vi "MergeMatchPoly.vi"(10 "Poly2D_2":T1, 11 "Poly2D_1":T1) -> (2 "Matched":bool, 3 "Poly2D":T1)   [LabVIEW 2014]
uses:
  TypeDefs/Poly2DwSlope.ctl
  TypeDefs/Point2DwSlope.ctl
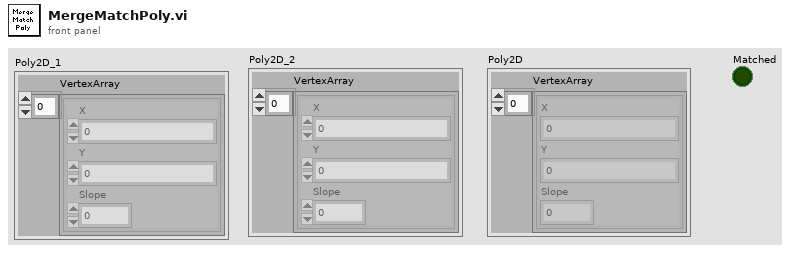
[diagram p1: front panel]
types:
  T1 = typedef "Poly2DwSlope.ctl" = cluster{"VertexArray":T2[]}
  T2 = typedef "Point2DwSlope.ctl" = cluster{"X":sgl, "Y":sgl, "Slope":dbl}
  T3 = enum16{"V1V1", "V1V2", "V2V1", "V2V2", "NoMatch"}
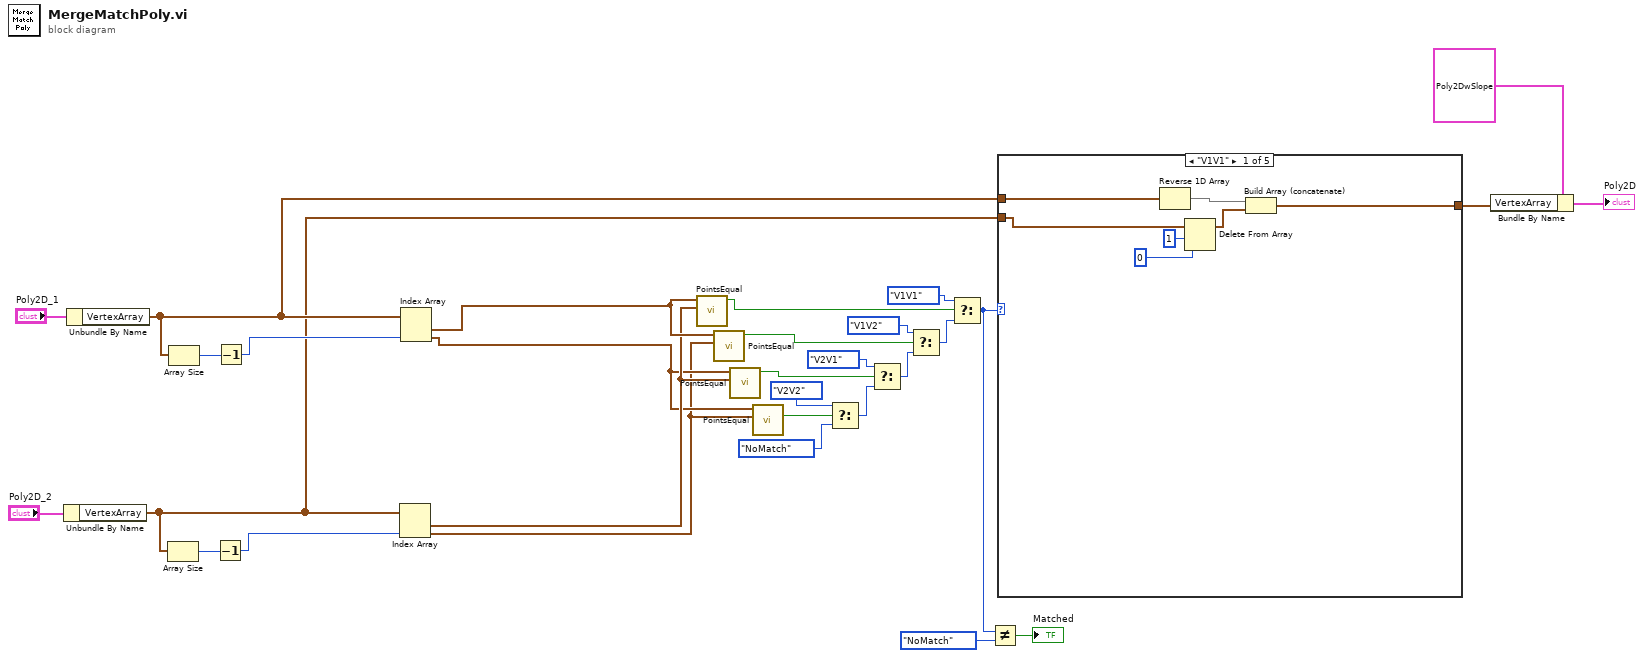
[diagram p0: block diagram]
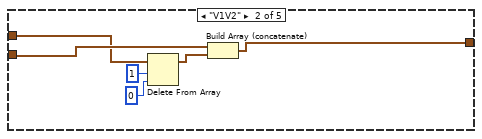
[diagram p2: hidden frame]
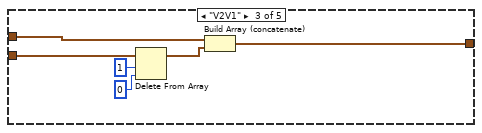
[diagram p3: hidden frame]
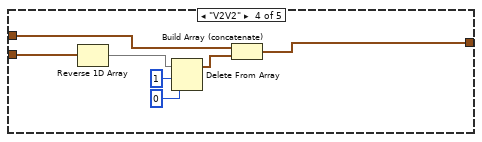
[diagram p4: hidden frame]
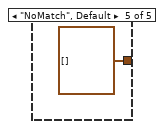
[diagram p5: hidden frame]
diagram:
  n1 = Unbundle By Name("Poly2D_2") -> ("VertexArray"=w12:T2[])
  n2 = Unbundle By Name("Poly2D_1") -> ("VertexArray"=w14:T2[])
  n3 = Array Size(array=w12) -> (size(s)=w27:i32)
  n4 = Array Size(array=w14) -> (size(s)=w30:i32)
  n5 = Decrement(x=w27) -> (x-1=w28:i32)
  n6 = Decrement(x=w30) -> (x-1=w29:i32)
  n7 = Index Array(array=w12, index #2=w28) -> (element #1=w5:T2, element #2=w2:T2)  [unwired: 1 in]
  n8 = Index Array(array=w14, index #2=w29) -> (element #1=w7:T2, element #2=w3:T2)  [unwired: 1 in]
  n9 = call "PointsEqual.vi"("Point2D_2"=w5, "Point2D_1"=w7) -> ("Equal?"=w8:bool)  [unwired: 9 in]
  n10 = call "PointsEqual.vi"("Point2D_2"=w2, "Point2D_1"=w7) -> ("Equal?"=w6:bool)  [unwired: 9 in]
  n11 = call "PointsEqual.vi"("Point2D_2"=w5, "Point2D_1"=w3) -> ("Equal?"=w4:bool)  [unwired: 9 in]
  n12 = call "PointsEqual.vi"("Point2D_2"=w2, "Point2D_1"=w3) -> ("Equal?"=w1:bool)  [unwired: 9 in]
  n13 = Select(t=T3."V2V2" ("f"), s=w1, f=T3."NoMatch") -> (s? t:f=w24:T3)
  n14 = Select(t=T3."V2V1" ("f"), s=w4, f=w24) -> (s? t:f=w25:T3)
  n15 = Select(t=T3."V1V2" ("f"), s=w6, f=w25) -> (s? t:f=w26:T3)
  n16 = Select(t=T3."V1V1" ("f"), s=w8, f=w26) -> (s? t:f=w18:T3)
  n17 = Not Equal?(x=w18, y=T3."NoMatch") -> (x != y?=→"Matched":bool)
  n18 = case shown="\"V1V1\"" w18 {
    tunnel: w14 -> [w37 w41 w49 w55 _]
    tunnel: w12 -> [w33 w42 w47 w56 _]
    tunnel: [w35 w43 w48 w54 T2[] []] -> w10
    frame "V1V1" {
      n19 = Reverse 1D Array(array=w37) -> (reversed array=w36:T2[])
      n20 = Delete From Array(array=w33, length=1, index=0) -> (array with subset deleted=w32:T2[])  [unwired: 1 out]
      n21 = Build Array (concatenate)(w36, w32) -> (w35:T2[])
    }
    frame "V1V2" {
      n22 = Delete From Array(array=w41, length=1, index=0) -> (array with subset deleted=w38:T2[])  [unwired: 1 out]
      n23 = Build Array (concatenate)(w42, w38) -> (w43:T2[])
    }
    frame "V2V1" {
      n24 = Delete From Array(array=w47, length=1, index=0) -> (array with subset deleted=w44:T2[])  [unwired: 1 out]
      n25 = Build Array (concatenate)(w49, w44) -> (w48:T2[])
    }
    frame "V2V2" {
      n26 = Reverse 1D Array(array=w56) -> (reversed array=w53:T2[])
      n27 = Delete From Array(array=w53, length=1, index=0) -> (array with subset deleted=w52:T2[])  [unwired: 1 out]
      n28 = Build Array (concatenate)(w55, w52) -> (w54:T2[])
    }
    frame "NoMatch", Default {
    }
  }
  n29 = Bundle By Name(cluster=T1 {"VertexArray"=[{"X"=8.830601, "Y"=7.172068, "Slope"=0.0}, {"X"=9.048535, "Y"=7.0468507, "Slope"=0.0}, {"X"=7.186762, "Y"=7.89218, "Slope"=0.0}, {"X"=7.186762, "Y"=7.89218, "Slope"=0.0}, {"X"=7.7402935, "Y"=7.713683, "Slope"=0.0}, {"X"=8.830601, "Y"=7.172068, "Slope"=0.0}, {"X"=8.385021, "Y"=7.4258633, "Slope"=0.0}, {"X"=7.7402935, "Y"=7.713683, "Slope"=0.0}, {"X"=9.932331, "Y"=6.418683, "Slope"=0.0}, {"X"=9.839655, "Y"=6.4924364, "Slope"=0.0}, {"X"=9.9016285, "Y"=6.443779, "Slope"=0.0}, {"X"=9.598942, "Y"=6.669884, "Slope"=0.0}, {"X"=9.440515, "Y"=6.776763, "Slope"=0.0}, {"X"=9.048535, "Y"=7.0468507, "Slope"=0.0}, {"X"=8.263897, "Y"=7.4805827, "Slope"=0.0}, {"X"=8.113029, "Y"=7.547746, "Slope"=0.0}, {"X"=8.385021, "Y"=7.4258633, "Slope"=0.0}, {"X"=-0.8597107, "Y"=6.3534126, "Slope"=0.0}, {"X"=-0.7344762, "Y"=6.2797923, "Slope"=0.0}, {"X"=-1.3683765, "Y"=6.656569, "Slope"=0.0}, {"X"=-1.5755129, "Y"=6.777237, "Slope"=0.0}, {"X"=-1.9615697, "Y"=6.9872913, "Slope"=0.0}, {"X"=-0.86309165, "Y"=6.3554897, "Slope"=0.0}, {"X"=0.7361049, "Y"=6.279792, "Slope"=0.0}, {"X"=0.7496544, "Y"=6.2877717, "Slope"=0.0}, {"X"=0.88590366, "Y"=6.367886, "Slope"=0.0}, {"X"=1.1839321, "Y"=6.5489907, "Slope"=0.0}, {"X"=1.7457985, "Y"=6.866745, "Slope"=0.0}, {"X"=1.6707515, "Y"=6.8289485, "Slope"=0.0}, {"X"=1.5142502, "Y"=6.7378664, "Slope"=0.0}, {"X"=1.5142502, "Y"=6.7378664, "Slope"=0.0}, {"X"=1.1839321, "Y"=6.5489907, "Slope"=0.0}, {"X"=0.88590366, "Y"=6.367886, "Slope"=0.0}, {"X"=0.8825039, "Y"=6.3658695, "Slope"=0.0}, {"X"=-9.596155, "Y"=6.670636, "Slope"=0.0}, {"X"=-9.82825, "Y"=6.4999356, "Slope"=0.0}, {"X"=-9.82825, "Y"=6.4999356, "Slope"=0.0}, {"X"=-9.930481, "Y"=6.418602, "Slope"=0.0}, {"X"=-8.38339, "Y"=7.4258623, "Slope"=0.0}, {"X"=-9.046905, "Y"=7.0468526, "Slope"=0.0}, {"X"=-9.439066, "Y"=6.7766366, "Slope"=0.0}, {"X"=-7.7386646, "Y"=7.7136784, "Slope"=0.0}, {"X"=-8.38339, "Y"=7.4258623, "Slope"=0.0}, {"X"=-7.185123, "Y"=7.89218, "Slope"=0.0}, {"X"=-7.439444, "Y"=7.8096337, "Slope"=0.0}, {"X"=-7.2370896, "Y"=7.874528, "Slope"=0.0}, {"X"=-7.113704, "Y"=7.913477, "Slope"=0.0}, {"X"=-7.6962314, "Y"=7.727286, "Slope"=0.0}, {"X"=5.3867097, "Y"=8.087741, "Slope"=0.0}, {"X"=5.732113, "Y"=8.092253, "Slope"=0.0}, {"X"=5.9348326, "Y"=8.090443, "Slope"=0.0}, {"X"=6.061366, "Y"=8.076636, "Slope"=0.0}, {"X"=6.061366, "Y"=8.076636, "Slope"=0.0}, {"X"=2.5593295, "Y"=7.295466, "Slope"=0.0}, {"X"=2.7117634, "Y"=7.365449, "Slope"=0.0}, {"X"=3.1518545, "Y"=7.5595336, "Slope"=0.0}, {"X"=3.387326, "Y"=7.651701, "Slope"=0.0}, {"X"=3.6230888, "Y"=7.737315, "Slope"=0.0}, {"X"=3.6230888, "Y"=7.737315, "Slope"=0.0}, {"X"=4.127137, "Y"=7.8904243, "Slope"=0.0}, {"X"=4.6575503, "Y"=8.007021, "Slope"=0.0}, {"X"=5.21036, "Y"=8.077528, "Slope"=0.0}, {"X"=4.851308, "Y"=8.034141, "Slope"=0.0}, {"X"=3.8247945, "Y"=7.7963767, "Slope"=0.0}, {"X"=4.3288827, "Y"=7.9346447, "Slope"=0.0}, {"X"=6.589266, "Y"=8.020231, "Slope"=0.0}, {"X"=6.589266, "Y"=8.020231, "Slope"=0.0}, {"X"=7.0844173, "Y"=7.9209275, "Slope"=0.0}, {"X"=7.1052027, "Y"=7.9160075, "Slope"=0.0}, {"X"=7.1153355, "Y"=7.9134755, "Slope"=0.0}, {"X"=11.066484, "Y"=5.9259615, "Slope"=0.0}, {"X"=11.296258, "Y"=5.921032, "Slope"=0.0}, {"X"=10.557279, "Y"=6.071126, "Slope"=0.0}, {"X"=10.38447, "Y"=6.147894, "Slope"=0.0}, {"X"=10.217855, "Y"=6.2337523, "Slope"=0.0}, {"X"=10.063343, "Y"=6.3245797, "Slope"=0.0}, {"X"=9.958954, "Y"=6.399936, "Slope"=0.0}, {"X"=11.366602, "Y"=6.3154464, "Slope"=0.0}, {"X"=11.3581505, "Y"=6.325527, "Slope"=0.0}, {"X"=11.381495, "Y"=5.947889, "Slope"=0.0}, {"X"=11.051102, "Y"=5.927362, "Slope"=0.0}, {"X"=11.428065, "Y"=6.2203074, "Slope"=0.0}, {"X"=11.366602, "Y"=6.3154464, "Slope"=0.0}, {"X"=11.4614525, "Y"=6.1327662, "Slope"=0.0}, {"X"=11.428065, "Y"=6.2203074, "Slope"=0.0}, {"X"=11.465086, "Y"=6.056186, "Slope"=0.0}, {"X"=11.4614525, "Y"=6.1327662, "Slope"=0.0}, {"X"=11.438299, "Y"=5.9936595, "Slope"=0.0}, {"X"=11.465086, "Y"=6.056186, "Slope"=0.0}, {"X"=11.438299, "Y"=5.9936595, "Slope"=0.0}, {"X"=11.354124, "Y"=5.938431, "Slope"=0.0}, {"X"=11.296258, "Y"=5.921032, "Slope"=0.0}, {"X"=11.185439, "Y"=5.914531, "Slope"=0.0}, {"X"=11.114248, "Y"=5.9222054, "Slope"=0.0}, {"X"=10.897281, "Y"=5.9582825, "Slope"=0.0}, {"X"=10.843447, "Y"=5.9742303, "Slope"=0.0}, {"X"=10.732583, "Y"=6.0081234, "Slope"=0.0}, {"X"=11.066484, "Y"=5.9259615, "Slope"=0.0}, {"X"=10.732583, "Y"=6.0081234, "Slope"=0.0}, {"X"=10.719951, "Y"=6.0130906, "Slope"=0.0}, {"X"=10.728581, "Y"=6.0096717, "Slope"=0.0}, {"X"=10.450941, "Y"=6.118535, "Slope"=0.0}, {"X"=10.289857, "Y"=6.1987867, "Slope"=0.0}, {"X"=10.174761, "Y"=6.259248, "Slope"=0.0}, {"X"=-0.3831223, "Y"=6.131223, "Slope"=0.0}, {"X"=-0.06600832, "Y"=6.079455, "Slope"=0.0}, {"X"=0.7361049, "Y"=6.279792, "Slope"=0.0}, {"X"=0.49233958, "Y"=6.1676245, "Slope"=0.0}, {"X"=0.41289893, "Y"=6.1388397, "Slope"=0.0}, {"X"=0.34931928, "Y"=6.1239376, "Slope"=0.0}, {"X"=0.06932907, "Y"=6.079732, "Slope"=0.0}, {"X"=0.06932907, "Y"=6.079732, "Slope"=0.0}, {"X"=-0.3457704, "Y"=6.1236205, "Slope"=0.0}, {"X"=-0.7011162, "Y"=6.2621675, "Slope"=0.0}, {"X"=-0.3831223, "Y"=6.131223, "Slope"=0.0}, {"X"=-0.7344762, "Y"=6.2797923, "Slope"=0.0}, {"X"=0.020335363, "Y"=6.074264, "Slope"=0.0}, {"X"=-2.5576975, "Y"=7.295468, "Slope"=0.0}, {"X"=-2.4127276, "Y"=7.2203803, "Slope"=0.0}, {"X"=-2.034087, "Y"=7.027823, "Slope"=0.0}, {"X"=-2.5576975, "Y"=7.295468, "Slope"=0.0}, {"X"=-2.9499915, "Y"=7.4758196, "Slope"=0.0}, {"X"=-2.7095613, "Y"=7.3651953, "Slope"=0.0}, {"X"=-5.784939, "Y"=8.094156, "Slope"=0.0}, {"X"=-5.5782948, "Y"=8.096169, "Slope"=0.0}, {"X"=-5.3852587, "Y"=8.087761, "Slope"=0.0}, {"X"=-5.208071, "Y"=8.077488, "Slope"=0.0}, {"X"=-5.208071, "Y"=8.077488, "Slope"=0.0}, {"X"=-3.3850975, "Y"=7.6514883, "Slope"=0.0}, {"X"=-3.150348, "Y"=7.5595837, "Slope"=0.0}, {"X"=-3.8916922, "Y"=7.821445, "Slope"=0.0}, {"X"=-3.6214588, "Y"=7.73732, "Slope"=0.0}, {"X"=-4.6554594, "Y"=8.006941, "Slope"=0.0}, {"X"=-4.327599, "Y"=7.934705, "Slope"=0.0}, {"X"=-4.1253557, "Y"=7.890371, "Slope"=0.0}, {"X"=-6.50035, "Y"=8.036642, "Slope"=0.0}, {"X"=-6.0605617, "Y"=8.076551, "Slope"=0.0}, {"X"=-5.933233, "Y"=8.090459, "Slope"=0.0}, {"X"=-7.0827866, "Y"=7.9209275, "Slope"=0.0}, {"X"=-6.5884337, "Y"=8.020078, "Slope"=0.0}, {"X"=-7.103572, "Y"=7.916008, "Slope"=0.0}, {"X"=-7.103572, "Y"=7.916008, "Slope"=0.0}, {"X"=1.9629927, "Y"=6.9872847, "Slope"=0.0}, {"X"=2.0286674, "Y"=7.024026, "Slope"=0.0}, {"X"=2.3005672, "Y"=7.166774, "Slope"=0.0}, {"X"=2.4886727, "Y"=7.2611537, "Slope"=0.0}, {"X"=2.5593295, "Y"=7.295466, "Slope"=0.0}, {"X"=2.2341883, "Y"=7.1319356, "Slope"=0.0}, {"X"=-11.046527, "Y"=5.9253874, "Slope"=0.0}, {"X"=-11.183571, "Y"=5.914618, "Slope"=0.0}, {"X"=-11.287836, "Y"=5.9220977, "Slope"=0.0}, {"X"=-10.211346, "Y"=6.231735, "Slope"=0.0}, {"X"=-10.551163, "Y"=6.075544, "Slope"=0.0}, {"X"=-10.033587, "Y"=6.345599, "Slope"=0.0}, {"X"=-10.211346, "Y"=6.231735, "Slope"=0.0}, {"X"=-10.033587, "Y"=6.345599, "Slope"=0.0}, {"X"=-10.060636, "Y"=6.324052, "Slope"=0.0}, {"X"=-11.438604, "Y"=5.9953485, "Slope"=0.0}, {"X"=-11.465441, "Y"=6.0578756, "Slope"=0.0}, {"X"=-11.428589, "Y"=6.222046, "Slope"=0.0}, {"X"=-11.369982, "Y"=6.305766, "Slope"=0.0}, {"X"=-11.363838, "Y"=6.3148956, "Slope"=0.0}, {"X"=-11.336758, "Y"=6.3461637, "Slope"=0.0}, {"X"=-11.306279, "Y"=5.9260035, "Slope"=0.0}, {"X"=-11.38179, "Y"=5.9495883, "Slope"=0.0}, {"X"=-11.417481, "Y"=6.239176, "Slope"=0.0}, {"X"=-11.363838, "Y"=6.3148956, "Slope"=0.0}, {"X"=-11.428589, "Y"=6.222046, "Slope"=0.0}, {"X"=-11.461873, "Y"=6.134476, "Slope"=0.0}, {"X"=-11.46389, "Y"=6.079863, "Slope"=0.0}, {"X"=-11.465441, "Y"=6.0578756, "Slope"=0.0}, {"X"=-11.438604, "Y"=5.9953485, "Slope"=0.0}, {"X"=-11.38179, "Y"=5.9495883, "Slope"=0.0}, {"X"=-11.251305, "Y"=5.9200234, "Slope"=0.0}, {"X"=-11.183571, "Y"=5.914618, "Slope"=0.0}, {"X"=-11.046527, "Y"=5.9253874, "Slope"=0.0}, {"X"=-10.892313, "Y"=5.956102, "Slope"=0.0}, {"X"=-10.892313, "Y"=5.956102, "Slope"=0.0}, {"X"=-10.557951, "Y"=6.072264, "Slope"=0.0}, {"X"=-10.56045, "Y"=6.071302, "Slope"=0.0}, {"X"=-10.727159, "Y"=6.0057144, "Slope"=0.0}, {"X"=-10.379647, "Y"=6.146689, "Slope"=0.0}, {"X"=-10.379647, "Y"=6.146689, "Slope"=0.0}, {"X"=10.444521, "Y"=7.162137, "Slope"=0.0}, {"X"=10.147654, "Y"=7.396959, "Slope"=0.0}, {"X"=11.135348, "Y"=6.5475297, "Slope"=0.0}, {"X"=10.8437395, "Y"=6.8065333, "Slope"=0.0}, {"X"=11.135348, "Y"=6.5475297, "Slope"=0.0}, {"X"=7.7880063, "Y"=8.844079, "Slope"=0.0}, {"X"=9.709546, "Y"=7.7424564, "Slope"=0.0}, {"X"=9.572357, "Y"=7.8359795, "Slope"=0.0}, {"X"=9.48678, "Y"=7.8936634, "Slope"=0.0}, {"X"=9.290509, "Y"=8.026892, "Slope"=0.0}, {"X"=8.41312, "Y"=8.549493, "Slope"=0.0}, {"X"=7.7880063, "Y"=8.844079, "Slope"=0.0}, {"X"=10.147654, "Y"=7.396959, "Slope"=0.0}, {"X"=8.9828415, "Y"=8.233359, "Slope"=0.0}, {"X"=9.290509, "Y"=8.026892, "Slope"=0.0}, {"X"=8.2803135, "Y"=8.623675, "Slope"=0.0}, {"X"=-10.352315, "Y"=7.234274, "Slope"=0.0}, {"X"=-10.44289, "Y"=7.162137, "Slope"=0.0}, {"X"=-9.570726, "Y"=7.8359795, "Slope"=0.0}, {"X"=-9.707915, "Y"=7.7424564, "Slope"=0.0}, {"X"=-10.352315, "Y"=7.234274, "Slope"=0.0}, {"X"=-7.7862473, "Y"=8.8441515, "Slope"=0.0}, {"X"=-8.180492, "Y"=8.666639, "Slope"=0.0}, {"X"=-8.678174, "Y"=8.404416, "Slope"=0.0}, {"X"=-8.24564, "Y"=8.638364, "Slope"=0.0}, {"X"=-8.278681, "Y"=8.623679, "Slope"=0.0}, {"X"=-8.678174, "Y"=8.404416, "Slope"=0.0}, {"X"=-9.570726, "Y"=7.8359795, "Slope"=0.0}, {"X"=-9.404453, "Y"=7.9493356, "Slope"=0.0}, {"X"=-9.108857, "Y"=8.149092, "Slope"=0.0}, {"X"=-9.288878, "Y"=8.026892, "Slope"=0.0}, {"X"=-11.273474, "Y"=6.4113665, "Slope"=0.0}, {"X"=-11.126271, "Y"=6.5544534, "Slope"=0.0}, {"X"=-10.842109, "Y"=6.8065333, "Slope"=0.0}, {"X"=-10.44289, "Y"=7.162137, "Slope"=0.0}, {"X"=-9.838867, "Y"=7.63992, "Slope"=0.0}, {"X"=-9.838867, "Y"=7.63992, "Slope"=0.0}, {"X"=-9.608428, "Y"=7.8105674, "Slope"=0.0}, {"X"=2.3092422, "Y"=9.555755, "Slope"=0.0}, {"X"=6.897631, "Y"=9.15439, "Slope"=0.0}, {"X"=6.9663086, "Y"=9.135237, "Slope"=0.0}, {"X"=6.826199, "Y"=9.173445, "Slope"=0.0}, {"X"=6.826199, "Y"=9.173445, "Slope"=0.0}, {"X"=6.8652363, "Y"=9.162923, "Slope"=0.0}, {"X"=7.4247684, "Y"=8.983244, "Slope"=0.0}, {"X"=7.478522, "Y"=8.961372, "Slope"=0.0}, {"X"=6.9663086, "Y"=9.135237, "Slope"=0.0}, {"X"=7.0981107, "Y"=9.089703, "Slope"=0.0}, {"X"=-7.0928435, "Y"=9.091241, "Slope"=0.0}, {"X"=-7.0928435, "Y"=9.091241, "Slope"=0.0}, {"X"=-7.476928, "Y"=8.961346, "Slope"=0.0}, {"X"=-7.4378753, "Y"=8.977723, "Slope"=0.0}, {"X"=-2.30762, "Y"=9.555743, "Slope"=0.0}, {"X"=-6.9646783, "Y"=9.135236, "Slope"=0.0}, {"X"=-6.8925557, "Y"=9.155159, "Slope"=0.0}, {"X"=6.644459, "Y"=9.217671, "Slope"=0.0}, {"X"=4.169504, "Y"=9.464814, "Slope"=0.0}, {"X"=3.7893963, "Y"=9.464789, "Slope"=0.0}, {"X"=3.404949, "Y"=9.4514675, "Slope"=0.0}, {"X"=5.0040536, "Y"=9.452098, "Slope"=0.0}, {"X"=3.0630891, "Y"=9.468226, "Slope"=0.0}, {"X"=3.0630891, "Y"=9.468226, "Slope"=0.0}, {"X"=2.724652, "Y"=9.495395, "Slope"=0.0}, {"X"=2.8233345, "Y"=9.493452, "Slope"=0.0}, {"X"=5.3548465, "Y"=9.425313, "Slope"=0.0}, {"X"=5.700839, "Y"=9.381838, "Slope"=0.0}, {"X"=6.4296727, "Y"=9.26174, "Slope"=0.0}, {"X"=6.644459, "Y"=9.217671, "Slope"=0.0}, {"X"=6.0274963, "Y"=9.334079, "Slope"=0.0}, {"X"=6.0274963, "Y"=9.334079, "Slope"=0.0}, {"X"=5.7321496, "Y"=9.377271, "Slope"=0.0}, {"X"=5.4556003, "Y"=9.414961, "Slope"=0.0}, {"X"=5.175468, "Y"=9.441919, "Slope"=0.0}, {"X"=4.65047, "Y"=9.461544, "Slope"=0.0}, {"X"=5.0040536, "Y"=9.452098, "Slope"=0.0}, {"X"=4.65047, "Y"=9.461544, "Slope"=0.0}, {"X"=4.607755, "Y"=9.461863, "Slope"=0.0}, {"X"=4.169504, "Y"=9.464814, "Slope"=0.0}, {"X"=3.7893963, "Y"=9.464789, "Slope"=0.0}, {"X"=3.404949, "Y"=9.4514675, "Slope"=0.0}, {"X"=-2.5918474, "Y"=9.499708, "Slope"=0.0}, {"X"=-2.7230513, "Y"=9.495405, "Slope"=0.0}, {"X"=-4.4270477, "Y"=9.454551, "Slope"=0.0}, {"X"=-4.618484, "Y"=9.458359, "Slope"=0.0}, {"X"=-5.072798, "Y"=9.436931, "Slope"=0.0}, {"X"=-6.491574, "Y"=9.240687, "Slope"=0.0}, {"X"=-6.7941, "Y"=9.181162, "Slope"=0.0}, {"X"=-4.618484, "Y"=9.458359, "Slope"=0.0}, {"X"=-3.0264053, "Y"=9.4683485, "Slope"=0.0}, {"X"=-3.0264053, "Y"=9.4683485, "Slope"=0.0}, {"X"=-3.2801545, "Y"=9.449338, "Slope"=0.0}, {"X"=-3.2801545, "Y"=9.449338, "Slope"=0.0}, {"X"=-3.5855074, "Y"=9.461267, "Slope"=0.0}, {"X"=-3.3309553, "Y"=9.444425, "Slope"=0.0}, {"X"=-3.9134116, "Y"=9.468681, "Slope"=0.0}, {"X"=-3.6864495, "Y"=9.468745, "Slope"=0.0}, {"X"=-4.239195, "Y"=9.465216, "Slope"=0.0}, {"X"=-4.1545463, "Y"=9.471141, "Slope"=0.0}, {"X"=-6.2067986, "Y"=9.297449, "Slope"=0.0}, {"X"=-5.920551, "Y"=9.346562, "Slope"=0.0}, {"X"=-5.639876, "Y"=9.383647, "Slope"=0.0}, {"X"=-5.3612723, "Y"=9.4128685, "Slope"=0.0}, {"X"=-5.0972753, "Y"=9.434096, "Slope"=0.0}, {"X"=-4.8120456, "Y"=9.44821, "Slope"=0.0}, {"X"=-6.2067986, "Y"=9.297449, "Slope"=0.0}, {"X"=-5.920551, "Y"=9.346562, "Slope"=0.0}, {"X"=-5.5172114, "Y"=9.401878, "Slope"=0.0}, {"X"=-5.8545833, "Y"=9.354088, "Slope"=0.0}, {"X"=2.2132256, "Y"=9.58271, "Slope"=0.0}, {"X"=1.8189816, "Y"=9.648704, "Slope"=0.0}, {"X"=1.8189816, "Y"=9.648704, "Slope"=0.0}, {"X"=2.2132256, "Y"=9.58271, "Slope"=0.0}, {"X"=-1.6634326, "Y"=9.665585, "Slope"=0.0}, {"X"=-1.8177922, "Y"=9.648689, "Slope"=0.0}, {"X"=-2.2115984, "Y"=9.582698, "Slope"=0.0}, {"X"=-1.9781245, "Y"=9.618462, "Slope"=0.0}, {"X"=0.72814083, "Y"=12.73701, "Slope"=0.0}, {"X"=-0.4196546, "Y"=12.743518, "Slope"=0.0}, {"X"=0.0007652063, "Y"=12.753558, "Slope"=0.0}, {"X"=0.5166687, "Y"=12.742718, "Slope"=0.0}, {"X"=0.4116929, "Y"=12.74487, "Slope"=0.0}, {"X"=1.0176144, "Y"=12.704265, "Slope"=0.0}, {"X"=1.4621797, "Y"=10.655392, "Slope"=0.0}, {"X"=1.5545752, "Y"=9.940707, "Slope"=0.0}, {"X"=1.4498512, "Y"=10.855028, "Slope"=0.0}, {"X"=1.4578543, "Y"=10.732892, "Slope"=0.0}, {"X"=1.5545752, "Y"=9.940707, "Slope"=0.0}, {"X"=1.6384071, "Y"=9.697788, "Slope"=0.0}, {"X"=1.6650634, "Y"=9.665521, "Slope"=0.0}, {"X"=1.5937715, "Y"=9.786305, "Slope"=0.0}, {"X"=1.5833964, "Y"=9.82258, "Slope"=0.0}, {"X"=1.4787083, "Y"=10.454523, "Slope"=0.0}, {"X"=1.4787083, "Y"=10.454523, "Slope"=0.0}, {"X"=1.5225716, "Y"=10.112019, "Slope"=0.0}, {"X"=1.5252, "Y"=10.098917, "Slope"=0.0}, {"X"=1.5426022, "Y"=10.012731, "Slope"=0.0}, {"X"=1.5040516, "Y"=10.237594, "Slope"=0.0}, {"X"=1.4989743, "Y"=10.272214, "Slope"=0.0}, {"X"=-1.6634326, "Y"=9.665585, "Slope"=0.0}, {"X"=-1.6236622, "Y"=9.727999, "Slope"=0.0}, {"X"=-1.5983242, "Y"=9.791381, "Slope"=0.0}, {"X"=-1.552802, "Y"=9.935697, "Slope"=0.0}, {"X"=-1.5983242, "Y"=9.791381, "Slope"=0.0}, {"X"=-1.5869727, "Y"=9.816154, "Slope"=0.0}, {"X"=-1.587823, "Y"=9.813162, "Slope"=0.0}, {"X"=-1.5209501, "Y"=10.100272, "Slope"=0.0}, {"X"=-1.4973384, "Y"=10.267358, "Slope"=0.0}, {"X"=-1.4585742, "Y"=10.705285, "Slope"=0.0}, {"X"=-1.4635025, "Y"=10.629503, "Slope"=0.0}, {"X"=-1.4770607, "Y"=10.45756, "Slope"=0.0}, {"X"=-1.4482204, "Y"=10.855038, "Slope"=0.0}, {"X"=-1.5474311, "Y"=9.963546, "Slope"=0.0}, {"X"=-1.4605238, "Y"=10.667121, "Slope"=0.0}, {"X"=-1.4973384, "Y"=10.267358, "Slope"=0.0}, {"X"=-1.3789781, "Y"=11.701954, "Slope"=0.0}, {"X"=-1.329632, "Y"=12.03006, "Slope"=0.0}, {"X"=-1.4286721, "Y"=11.182402, "Slope"=0.0}, {"X"=-1.0699232, "Y"=12.697788, "Slope"=0.0}, {"X"=-1.0901189, "Y"=12.68052, "Slope"=0.0}, {"X"=-1.1646048, "Y"=12.571568, "Slope"=0.0}, {"X"=-1.2407196, "Y"=12.380032, "Slope"=0.0}, {"X"=-1.2720493, "Y"=12.2814455, "Slope"=0.0}, {"X"=-1.0159835, "Y"=12.704266, "Slope"=0.0}, {"X"=-1.3427985, "Y"=11.95073, "Slope"=0.0}, {"X"=-1.4286721, "Y"=11.182402, "Slope"=0.0}, {"X"=-1.4014932, "Y"=11.485938, "Slope"=0.0}, {"X"=-1.4188328, "Y"=11.319262, "Slope"=0.0}, {"X"=-1.2407196, "Y"=12.380032, "Slope"=0.0}, {"X"=-1.1646048, "Y"=12.571568, "Slope"=0.0}, {"X"=-1.0901189, "Y"=12.68052, "Slope"=0.0}, {"X"=1.1517563, "Y"=12.598272, "Slope"=0.0}, {"X"=1.04348, "Y"=12.704147, "Slope"=0.0}, {"X"=1.0855013, "Y"=12.679428, "Slope"=0.0}, {"X"=1.2149384, "Y"=12.468784, "Slope"=0.0}, {"X"=1.1729327, "Y"=12.554751, "Slope"=0.0}, {"X"=1.1517563, "Y"=12.598272, "Slope"=0.0}, {"X"=1.3806208, "Y"=11.686752, "Slope"=0.0}, {"X"=1.4204677, "Y"=11.315399, "Slope"=0.0}, {"X"=1.4296497, "Y"=11.192336, "Slope"=0.0}, {"X"=1.4498512, "Y"=10.855028, "Slope"=0.0}, {"X"=1.3312752, "Y"=12.016102, "Slope"=0.0}, {"X"=1.3806208, "Y"=11.686752, "Slope"=0.0}, {"X"=1.2736847, "Y"=12.293916, "Slope"=0.0}, {"X"=1.2751907, "Y"=12.2876835, "Slope"=0.0}, {"X"=1.3312752, "Y"=12.016102, "Slope"=0.0}, {"X"=1.2740316, "Y"=12.292477, "Slope"=0.0}, {"X"=1.2736847, "Y"=12.293916, "Slope"=0.0}, {"X"=1.1150376, "Y"=12.643135, "Slope"=0.0}, {"X"=-12.02701, "Y"=-8.883595, "Slope"=0.0}, {"X"=-11.930874, "Y"=-8.755775, "Slope"=0.0}, {"X"=-12.135208, "Y"=-9.147686, "Slope"=0.0}, {"X"=-12.100296, "Y"=-9.031299, "Slope"=0.0}, {"X"=-12.095111, "Y"=-9.902619, "Slope"=0.0}, {"X"=-12.067877, "Y"=-9.970935, "Slope"=0.0}, {"X"=-12.029266, "Y"=-10.067103, "Slope"=0.0}, {"X"=-12.029266, "Y"=-10.067103, "Slope"=0.0}, {"X"=-11.9856825, "Y"=-10.148499, "Slope"=0.0}, {"X"=-12.142309, "Y"=-9.728694, "Slope"=0.0}, {"X"=-12.127801, "Y"=-9.782524, "Slope"=0.0}, {"X"=-12.1486845, "Y"=-9.194613, "Slope"=0.0}, {"X"=-12.170822, "Y"=-9.369725, "Slope"=0.0}, {"X"=-12.1705885, "Y"=-9.389268, "Slope"=0.0}, {"X"=-12.168238, "Y"=-9.549478, "Slope"=0.0}, {"X"=-12.168238, "Y"=-9.549478, "Slope"=0.0}, {"X"=-11.8144655, "Y"=-8.65208, "Slope"=0.0}, {"X"=-11.7577095, "Y"=-8.616993, "Slope"=0.0}, {"X"=-11.8144655, "Y"=-8.65208, "Slope"=0.0}, {"X"=-12.02701, "Y"=-8.883595, "Slope"=0.0}, {"X"=-12.016741, "Y"=-8.869859, "Slope"=0.0}, {"X"=-12.135208, "Y"=-9.147686, "Slope"=0.0}, {"X"=-11.294352, "Y"=-10.777359, "Slope"=0.0}, {"X"=-11.318705, "Y"=-10.768083, "Slope"=0.0}, {"X"=-11.894479, "Y"=-10.297557, "Slope"=0.0}, {"X"=-11.864539, "Y"=-10.3413925, "Slope"=0.0}, {"X"=-11.542754, "Y"=-10.650674, "Slope"=0.0}, {"X"=-11.322815, "Y"=-10.765945, "Slope"=0.0}, {"X"=-11.660817, "Y"=-10.56013, "Slope"=0.0}, {"X"=-11.684228, "Y"=-10.5376215, "Slope"=0.0}, {"X"=-11.768559, "Y"=-10.456095, "Slope"=0.0}, {"X"=-11.768559, "Y"=-10.456095, "Slope"=0.0}, {"X"=-11.318705, "Y"=-10.768083, "Slope"=0.0}, {"X"=-11.864539, "Y"=-10.3413925, "Slope"=0.0}, {"X"=-11.569865, "Y"=-8.037169, "Slope"=0.0}, {"X"=-11.563985, "Y"=-8.070403, "Slope"=0.0}, {"X"=-11.552345, "Y"=-8.164364, "Slope"=0.0}, {"X"=-11.553843, "Y"=-8.257444, "Slope"=0.0}, {"X"=-11.568527, "Y"=-8.345382, "Slope"=0.0}, {"X"=-11.595686, "Y"=-8.425903, "Slope"=0.0}, {"X"=-11.632769, "Y"=-8.4943, "Slope"=0.0}, {"X"=-11.679456, "Y"=-8.552723, "Slope"=0.0}, {"X"=-11.734429, "Y"=-8.599825, "Slope"=0.0}, {"X"=-11.700265, "Y"=-8.574736, "Slope"=0.0}, {"X"=-11.650671, "Y"=-8.521496, "Slope"=0.0}, {"X"=-11.61017, "Y"=-8.45847, "Slope"=0.0}, {"X"=-11.579652, "Y"=-8.387263, "Slope"=0.0}, {"X"=-11.558998, "Y"=-8.305826, "Slope"=0.0}, {"X"=-11.550331, "Y"=-8.218866, "Slope"=0.0}, {"X"=-11.553987, "Y"=-8.128481, "Slope"=0.0}, {"X"=-11.3296585, "Y"=-13.300342, "Slope"=0.0}, {"X"=-11.256834, "Y"=-13.179006, "Slope"=0.0}, {"X"=-11.151226, "Y"=-13.057631, "Slope"=0.0}, {"X"=-11.16577, "Y"=-13.070827, "Slope"=0.0}, {"X"=-11.1825075, "Y"=-13.090706, "Slope"=0.0}, {"X"=-11.051586, "Y"=-12.9728775, "Slope"=0.0}, {"X"=-11.051586, "Y"=-12.9728775, "Slope"=0.0}, {"X"=-10.939525, "Y"=-12.903137, "Slope"=0.0}, {"X"=-10.939525, "Y"=-12.903137, "Slope"=0.0}, {"X"=-10.849801, "Y"=-14.563225, "Slope"=0.0}, {"X"=-11.164953, "Y"=-14.337027, "Slope"=0.0}, {"X"=-11.067114, "Y"=-14.428592, "Slope"=0.0}, {"X"=-11.141206, "Y"=-14.359256, "Slope"=0.0}, {"X"=-11.164953, "Y"=-14.337027, "Slope"=0.0}, {"X"=-10.933373, "Y"=-14.519123, "Slope"=0.0}, {"X"=-10.960547, "Y"=-14.504524, "Slope"=0.0}, {"X"=-11.250185, "Y"=-14.232005, "Slope"=0.0}, {"X"=-11.421939, "Y"=-13.710416, "Slope"=0.0}, {"X"=-11.408769, "Y"=-13.850409, "Slope"=0.0}, {"X"=-11.419471, "Y"=-13.73668, "Slope"=0.0}, {"X"=-11.421939, "Y"=-13.710416, "Slope"=0.0}, {"X"=-11.413157, "Y"=-13.569632, "Slope"=0.0}, {"X"=-11.382209, "Y"=-13.431717, "Slope"=0.0}, {"X"=-11.387743, "Y"=-13.456368, "Slope"=0.0}, {"X"=-11.256834, "Y"=-13.179006, "Slope"=0.0}, {"X"=-11.26992, "Y"=-13.200806, "Slope"=0.0}, {"X"=-11.321019, "Y"=-14.114156, "Slope"=0.0}, {"X"=-11.305685, "Y"=-14.139672, "Slope"=0.0}, {"X"=-11.413157, "Y"=-13.569632, "Slope"=0.0}, {"X"=-11.402093, "Y"=-13.876914, "Slope"=0.0}, {"X"=-11.374592, "Y"=-13.986052, "Slope"=0.0}, {"X"=-11.250185, "Y"=-14.232005, "Slope"=0.0}, {"X"=-11.913404, "Y"=-6.6864777, "Slope"=0.0}, {"X"=-11.797986, "Y"=-7.147725, "Slope"=0.0}, {"X"=-12.13859, "Y"=-5.825948, "Slope"=0.0}, {"X"=-11.913404, "Y"=-6.6864777, "Slope"=0.0}, {"X"=-12.225317, "Y"=-5.519531, "Slope"=0.0}, {"X"=-12.225317, "Y"=-5.519531, "Slope"=0.0}, {"X"=-11.221693, "Y"=-10.810644, "Slope"=0.0}, {"X"=-11.294352, "Y"=-10.777359, "Slope"=0.0}, {"X"=-11.030285, "Y"=-10.970268, "Slope"=0.0}, {"X"=-11.091174, "Y"=-10.905559, "Slope"=0.0}, {"X"=-11.160064, "Y"=-10.849495, "Slope"=0.0}, {"X"=-11.152487, "Y"=-10.854256, "Slope"=0.0}, {"X"=-10.860488, "Y"=-11.333081, "Slope"=0.0}, {"X"=-10.880931, "Y"=-11.255504, "Slope"=0.0}, {"X"=-10.892451, "Y"=-11.2184515, "Slope"=0.0}, {"X"=-10.922376, "Y"=-11.142319, "Slope"=0.0}, {"X"=-10.928037, "Y"=-11.131481, "Slope"=0.0}, {"X"=-10.928037, "Y"=-11.131481, "Slope"=0.0}, {"X"=-10.970161, "Y"=-11.053841, "Slope"=0.0}, {"X"=-11.02817, "Y"=-10.972571, "Slope"=0.0}, {"X"=-10.973595, "Y"=-11.048819, "Slope"=0.0}, {"X"=-11.028286, "Y"=-10.97244, "Slope"=0.0}, {"X"=-11.087512, "Y"=-10.908614, "Slope"=0.0}, {"X"=-10.665473, "Y"=-12.46586, "Slope"=0.0}, {"X"=-10.664033, "Y"=-12.508651, "Slope"=0.0}, {"X"=-10.673386, "Y"=-12.582449, "Slope"=0.0}, {"X"=-10.694738, "Y"=-12.653376, "Slope"=0.0}, {"X"=-10.72751, "Y"=-12.7196455, "Slope"=0.0}, {"X"=-10.768068, "Y"=-12.776132, "Slope"=0.0}, {"X"=-10.816997, "Y"=-12.825721, "Slope"=0.0}, {"X"=-10.902442, "Y"=-12.882612, "Slope"=0.0}, {"X"=-10.916191, "Y"=-12.891214, "Slope"=0.0}, {"X"=-10.800756, "Y"=-12.811512, "Slope"=0.0}, {"X"=-10.754254, "Y"=-12.759442, "Slope"=0.0}, {"X"=-10.716546, "Y"=-12.700924, "Slope"=0.0}, {"X"=-10.686941, "Y"=-12.633139, "Slope"=0.0}, {"X"=-10.668956, "Y"=-12.561274, "Slope"=0.0}, {"X"=-10.663047, "Y"=-12.487158, "Slope"=0.0}, {"X"=-10.665473, "Y"=-12.46586, "Slope"=0.0}, {"X"=-10.710455, "Y"=-14.615379, "Slope"=0.0}, {"X"=-10.849801, "Y"=-14.563225, "Slope"=0.0}, {"X"=-10.848216, "Y"=-14.563806, "Slope"=0.0}, {"X"=-10.7669525, "Y"=-14.595915, "Slope"=0.0}, {"X"=-10.30013, "Y"=-14.642541, "Slope"=0.0}, {"X"=-10.446137, "Y"=-14.654243, "Slope"=0.0}, {"X"=-10.446137, "Y"=-14.654243, "Slope"=0.0}, {"X"=-10.563266, "Y"=-14.646091, "Slope"=0.0}, {"X"=-10.469295, "Y"=-14.651767, "Slope"=0.0}, {"X"=-9.648653, "Y"=-14.927292, "Slope"=0.0}, {"X"=-9.645592, "Y"=-14.928906, "Slope"=0.0}, {"X"=-9.606909, "Y"=-14.948134, "Slope"=0.0}, {"X"=-9.606909, "Y"=-14.948134, "Slope"=0.0}, {"X"=-9.846963, "Y"=-14.788051, "Slope"=0.0}, {"X"=-9.851051, "Y"=-14.785206, "Slope"=0.0}, {"X"=-9.854066, "Y"=-14.783052, "Slope"=0.0}, {"X"=-9.772256, "Y"=-14.849932, "Slope"=0.0}, {"X"=-9.772256, "Y"=-14.849932, "Slope"=0.0}, {"X"=-9.739692, "Y"=-14.872915, "Slope"=0.0}, {"X"=-9.722611, "Y"=-14.884181, "Slope"=0.0}, {"X"=-9.722611, "Y"=-14.884181, "Slope"=0.0}, {"X"=-9.686776, "Y"=-14.906165, "Slope"=0.0}, {"X"=-12.650918, "Y"=-3.9329345, "Slope"=0.0}, {"X"=-12.648346, "Y"=-3.8170426, "Slope"=0.0}, {"X"=-12.631214, "Y"=-3.735219, "Slope"=0.0}, {"X"=-12.623239, "Y"=-3.7092106, "Slope"=0.0}, {"X"=-12.623239, "Y"=-3.7092106, "Slope"=0.0}, {"X"=-12.62978, "Y"=-4.049288, "Slope"=0.0}, {"X"=-12.650918, "Y"=-3.9329345, "Slope"=0.0}, {"X"=-12.57752, "Y"=-3.6137216, "Slope"=0.0}, {"X"=-12.57752, "Y"=-3.6137216, "Slope"=0.0}, {"X"=-12.513479, "Y"=-3.534193, "Slope"=0.0}, {"X"=-12.513479, "Y"=-3.534193, "Slope"=0.0}, {"X"=-12.433673, "Y"=-3.4738154, "Slope"=0.0}, {"X"=-12.433673, "Y"=-3.4738154, "Slope"=0.0}, {"X"=-12.357601, "Y"=-3.4377882, "Slope"=0.0}, {"X"=-12.340974, "Y"=-3.43551, "Slope"=0.0}, {"X"=-3.3543682, "Y"=-1.112888, "Slope"=0.0}, {"X"=-3.2291064, "Y"=-0.992266, "Slope"=0.0}, {"X"=-2.9242365, "Y"=-0.58080864, "Slope"=0.0}, {"X"=-3.0170414, "Y"=-0.7281756, "Slope"=0.0}, {"X"=-3.2999249, "Y"=-1.0642368, "Slope"=0.0}, {"X"=-3.4399374, "Y"=-1.1873536, "Slope"=0.0}, {"X"=-3.0855627, "Y"=-0.82208127, "Slope"=0.0}, {"X"=-3.0855627, "Y"=-0.82208127, "Slope"=0.0}, {"X"=-10.675578, "Y"=-12.364202, "Slope"=0.0}, {"X"=-10.771004, "Y"=-11.824437, "Slope"=0.0}, {"X"=-10.784014, "Y"=-11.759393, "Slope"=0.0}, {"X"=-10.784014, "Y"=-11.759393, "Slope"=0.0}, {"X"=-5.6554403, "Y"=5.9907885, "Slope"=0.0}, {"X"=-4.815982, "Y"=7.0489526, "Slope"=0.0}, {"X"=-4.849929, "Y"=6.9179187, "Slope"=0.0}, {"X"=-5.0451655, "Y"=6.464496, "Slope"=0.0}, {"X"=-5.2916584, "Y"=6.1826806, "Slope"=0.0}, {"X"=-5.162795, "Y"=6.294174, "Slope"=0.0}, {"X"=-5.543999, "Y"=6.0281105, "Slope"=0.0}, {"X"=-6.3306594, "Y"=6.0232587, "Slope"=0.0}, {"X"=-6.6277933, "Y"=6.1670747, "Slope"=0.0}, {"X"=-6.934379, "Y"=6.406201, "Slope"=0.0}, {"X"=-6.8160934, "Y"=6.3108954, "Slope"=0.0}, {"X"=-6.4554677, "Y"=6.0813403, "Slope"=0.0}, {"X"=-6.3306594, "Y"=6.0232587, "Slope"=0.0}, {"X"=-6.250035, "Y"=6.003523, "Slope"=0.0}, {"X"=-5.8642983, "Y"=5.95157, "Slope"=0.0}, {"X"=-5.6554403, "Y"=5.9907885, "Slope"=0.0}, {"X"=-5.924631, "Y"=5.951281, "Slope"=0.0}, {"X"=-4.849929, "Y"=6.9179187, "Slope"=0.0}, {"X"=-5.0451655, "Y"=6.464496, "Slope"=0.0}, {"X"=-10.292118, "Y"=-14.642107, "Slope"=0.0}, {"X"=-10.171297, "Y"=-14.638529, "Slope"=0.0}, {"X"=-10.041175, "Y"=-14.666001, "Slope"=0.0}, {"X"=-10.041588, "Y"=-14.665805, "Slope"=0.0}, {"X"=-10.162641, "Y"=-14.639628, "Slope"=0.0}, {"X"=-10.162641, "Y"=-14.639628, "Slope"=0.0}, {"X"=-10.164488, "Y"=-14.639059, "Slope"=0.0}, {"X"=-10.166433, "Y"=-14.638672, "Slope"=0.0}, {"X"=-9.460867, "Y"=-15.017409, "Slope"=0.0}, {"X"=-9.437974, "Y"=-15.031419, "Slope"=0.0}, {"X"=-9.437974, "Y"=-15.031419, "Slope"=0.0}, {"X"=-9.564893, "Y"=-14.966767, "Slope"=0.0}, {"X"=-9.525483, "Y"=-14.983645, "Slope"=0.0}, {"X"=-9.505892, "Y"=-14.993372, "Slope"=0.0}, {"X"=-9.58607, "Y"=-14.956815, "Slope"=0.0}, {"X"=-9.854066, "Y"=-14.783052, "Slope"=0.0}, {"X"=-9.884875, "Y"=-14.755914, "Slope"=0.0}, {"X"=-9.887594, "Y"=-14.7537775, "Slope"=0.0}, {"X"=-9.901564, "Y"=-14.742871, "Slope"=0.0}, {"X"=-9.548078, "Y"=-14.973137, "Slope"=0.0}, {"X"=-3.9709668, "Y"=0.83104026, "Slope"=0.0}, {"X"=-3.793563, "Y"=0.96303296, "Slope"=0.0}, {"X"=-3.6569257, "Y"=1.1055839, "Slope"=0.0}, {"X"=-3.5894172, "Y"=1.7002168, "Slope"=0.0}, {"X"=-6.403721, "Y"=1.1754698, "Slope"=0.0}, {"X"=-6.3508883, "Y"=1.1123196, "Slope"=0.0}, {"X"=-6.3508883, "Y"=1.1123196, "Slope"=0.0}, {"X"=-3.8743422, "Y"=0.89098823, "Slope"=0.0}, {"X"=-3.673383, "Y"=1.0765003, "Slope"=0.0}, {"X"=-4.5997987, "Y"=2.4074922, "Slope"=0.0}, {"X"=-4.870421, "Y"=2.4419749, "Slope"=0.0}, {"X"=-5.4179683, "Y"=2.447132, "Slope"=0.0}, {"X"=-5.843843, "Y"=2.364739, "Slope"=0.0}, {"X"=-6.137103, "Y"=2.2173433, "Slope"=0.0}, {"X"=-4.5921416, "Y"=0.6193031, "Slope"=0.0}, {"X"=-4.246321, "Y"=0.71311134, "Slope"=0.0}, {"X"=-4.470907, "Y"=0.6456365, "Slope"=0.0}, {"X"=-5.0984373, "Y"=0.6077611, "Slope"=0.0}, {"X"=-5.0984373, "Y"=0.6077611, "Slope"=0.0}, {"X"=-4.658153, "Y"=0.60572743, "Slope"=0.0}, {"X"=-5.2277637, "Y"=0.60893834, "Slope"=0.0}, {"X"=-5.792988, "Y"=0.74757576, "Slope"=0.0}, {"X"=-6.1827035, "Y"=0.97466177, "Slope"=0.0}, {"X"=-4.0832763, "Y"=0.7651222, "Slope"=0.0}, {"X"=-3.5581236, "Y"=1.3308722, "Slope"=0.0}, {"X"=-3.5581236, "Y"=1.3308722, "Slope"=0.0}, {"X"=-3.562323, "Y"=1.6246175, "Slope"=0.0}, {"X"=-6.4372854, "Y"=1.2494335, "Slope"=0.0}, {"X"=-6.532556, "Y"=1.6240577, "Slope"=0.0}, {"X"=-6.472267, "Y"=1.8649976, "Slope"=0.0}, {"X"=-6.358427, "Y"=2.0599158, "Slope"=0.0}, {"X"=-3.5492315, "Y"=1.3571573, "Slope"=0.0}, {"X"=-6.535462, "Y"=1.4654024, "Slope"=0.0}, {"X"=-3.5894172, "Y"=1.7002168, "Slope"=0.0}, {"X"=-6.53032, "Y"=1.7503738, "Slope"=0.0}, {"X"=-4.0369825, "Y"=2.1945257, "Slope"=0.0}, {"X"=-4.0369825, "Y"=2.1945257, "Slope"=0.0}, {"X"=-6.137103, "Y"=2.2173433, "Slope"=0.0}, {"X"=-6.3882627, "Y"=2.0303822, "Slope"=0.0}, {"X"=-4.870421, "Y"=2.4419749, "Slope"=0.0}, {"X"=-5.4179683, "Y"=2.447132, "Slope"=0.0}, {"X"=-5.843843, "Y"=2.364739, "Slope"=0.0}, {"X"=-6.7040663, "Y"=7.639021, "Slope"=0.0}, {"X"=-6.676446, "Y"=7.650669, "Slope"=0.0}, {"X"=-4.9156322, "Y"=7.482542, "Slope"=0.0}, {"X"=-4.855164, "Y"=7.3850617, "Slope"=0.0}, {"X"=-4.815982, "Y"=7.0489526, "Slope"=0.0}, {"X"=-4.8155766, "Y"=7.1894574, "Slope"=0.0}, {"X"=-4.8181634, "Y"=7.2813587, "Slope"=0.0}, {"X"=-5.878805, "Y"=7.82959, "Slope"=0.0}, {"X"=-5.5302444, "Y"=7.8090086, "Slope"=0.0}, {"X"=-5.289001, "Y"=7.740003, "Slope"=0.0}, {"X"=-6.215815, "Y"=7.7961473, "Slope"=0.0}, {"X"=-5.11955, "Y"=7.66165, "Slope"=0.0}, {"X"=-5.0015216, "Y"=7.5747905, "Slope"=0.0}, {"X"=-6.215815, "Y"=7.7961473, "Slope"=0.0}, {"X"=-5.878805, "Y"=7.82959, "Slope"=0.0}, {"X"=-5.5302444, "Y"=7.8090086, "Slope"=0.0}, {"X"=-5.289001, "Y"=7.740003, "Slope"=0.0}, {"X"=-5.0015216, "Y"=7.5747905, "Slope"=0.0}, {"X"=-4.978973, "Y"=7.5499973, "Slope"=0.0}, {"X"=-5.11955, "Y"=7.66165, "Slope"=0.0}, {"X"=-4.855164, "Y"=7.3850617, "Slope"=0.0}, {"X"=-6.8678813, "Y"=7.52537, "Slope"=0.0}, {"X"=-6.777728, "Y"=7.5995193, "Slope"=0.0}, {"X"=-6.856725, "Y"=7.5351534, "Slope"=0.0}, {"X"=-6.8603616, "Y"=7.531958, "Slope"=0.0}, {"X"=-6.875995, "Y"=7.5181913, "Slope"=0.0}, {"X"=-6.888495, "Y"=7.503174, "Slope"=0.0}, {"X"=-6.888495, "Y"=7.503174, "Slope"=0.0}, {"X"=-6.818737, "Y"=7.5675063, "Slope"=0.0}, {"X"=-6.7040663, "Y"=7.639021, "Slope"=0.0}, {"X"=-6.777728, "Y"=7.5995193, "Slope"=0.0}, {"X"=-6.84122, "Y"=7.5485497, "Slope"=0.0}, {"X"=-6.8429217, "Y"=7.5470734, "Slope"=0.0}, {"X"=-6.8310695, "Y"=7.5571713, "Slope"=0.0}, {"X"=-6.875995, "Y"=7.5181913, "Slope"=0.0}, {"X"=-6.8678813, "Y"=7.52537, "Slope"=0.0}, {"X"=-6.818737, "Y"=7.5675063, "Slope"=0.0}, {"X"=-6.822014, "Y"=7.5647697, "Slope"=0.0}, {"X"=-7.0596285, "Y"=6.551442, "Slope"=0.0}, {"X"=-7.091569, "Y"=7.302365, "Slope"=0.0}, {"X"=-7.0596285, "Y"=6.551442, "Slope"=0.0}, {"X"=-7.1912403, "Y"=6.921647, "Slope"=0.0}, {"X"=-7.155486, "Y"=7.136137, "Slope"=0.0}, {"X"=-7.200834, "Y"=7.019425, "Slope"=0.0}, {"X"=-6.894214, "Y"=7.488816, "Slope"=0.0}, {"X"=-7.065946, "Y"=7.3290687, "Slope"=0.0}, {"X"=-7.086213, "Y"=7.308606, "Slope"=0.0}, {"X"=-7.1912403, "Y"=6.921647, "Slope"=0.0}, {"X"=-10.025236, "Y"=-14.673826, "Slope"=0.0}, {"X"=-9.951885, "Y"=-14.708637, "Slope"=0.0}, {"X"=-9.932256, "Y"=-14.721165, "Slope"=0.0}, {"X"=-9.319345, "Y"=-15.105489, "Slope"=0.0}, {"X"=-8.93562, "Y"=-15.3406515, "Slope"=0.0}, {"X"=-9.265467, "Y"=-15.138879, "Slope"=0.0}, {"X"=-9.319345, "Y"=-15.105489, "Slope"=0.0}, {"X"=-8.488454, "Y"=-15.60559, "Slope"=0.0}, {"X"=-8.50379, "Y"=-15.596214, "Slope"=0.0}, {"X"=-8.0269165, "Y"=-15.876325, "Slope"=0.0}, {"X"=-7.546262, "Y"=-16.157545, "Slope"=0.0}, {"X"=-7.6811376, "Y"=-16.072777, "Slope"=0.0}, {"X"=-8.93562, "Y"=-15.3406515, "Slope"=0.0}, {"X"=-8.50379, "Y"=-15.596214, "Slope"=0.0}, {"X"=-8.488454, "Y"=-15.60559, "Slope"=0.0}, {"X"=-7.546262, "Y"=-16.157545, "Slope"=0.0}, {"X"=-7.4288588, "Y"=-16.223211, "Slope"=0.0}, {"X"=-7.2701726, "Y"=-16.31386, "Slope"=0.0}, {"X"=12.028641, "Y"=-8.883595, "Slope"=0.0}, {"X"=11.803545, "Y"=-8.642787, "Slope"=0.0}, {"X"=11.75934, "Y"=-8.616993, "Slope"=0.0}, {"X"=11.932505, "Y"=-8.755775, "Slope"=0.0}, {"X"=11.945703, "Y"=-8.773437, "Slope"=0.0}, {"X"=12.149438, "Y"=-9.191597, "Slope"=0.0}, {"X"=12.150315, "Y"=-9.194613, "Slope"=0.0}, {"X"=12.172453, "Y"=-9.369725, "Slope"=0.0}, {"X"=12.169868, "Y"=-9.549478, "Slope"=0.0}, {"X"=11.987313, "Y"=-10.148499, "Slope"=0.0}, {"X"=12.096742, "Y"=-9.902619, "Slope"=0.0}, {"X"=12.030897, "Y"=-10.067103, "Slope"=0.0}, {"X"=11.987313, "Y"=-10.148499, "Slope"=0.0}, {"X"=12.14394, "Y"=-9.728694, "Slope"=0.0}, {"X"=11.816096, "Y"=-8.65208, "Slope"=0.0}, {"X"=12.028641, "Y"=-8.883595, "Slope"=0.0}, {"X"=12.101927, "Y"=-9.031299, "Slope"=0.0}, {"X"=12.104113, "Y"=-9.038665, "Slope"=0.0}, {"X"=12.136839, "Y"=-9.147686, "Slope"=0.0}, {"X"=12.150315, "Y"=-9.194613, "Slope"=0.0}, {"X"=12.172453, "Y"=-9.369725, "Slope"=0.0}, {"X"=12.169868, "Y"=-9.549478, "Slope"=0.0}, {"X"=12.14394, "Y"=-9.728694, "Slope"=0.0}, {"X"=12.096742, "Y"=-9.902619, "Slope"=0.0}, {"X"=11.571496, "Y"=-8.037169, "Slope"=0.0}, {"X"=11.555617, "Y"=-8.128481, "Slope"=0.0}, {"X"=11.555617, "Y"=-8.128481, "Slope"=0.0}, {"X"=11.551962, "Y"=-8.218866, "Slope"=0.0}, {"X"=11.560629, "Y"=-8.305826, "Slope"=0.0}, {"X"=11.581283, "Y"=-8.387263, "Slope"=0.0}, {"X"=11.611801, "Y"=-8.45847, "Slope"=0.0}, {"X"=11.652302, "Y"=-8.521496, "Slope"=0.0}, {"X"=11.701896, "Y"=-8.574736, "Slope"=0.0}, {"X"=11.73606, "Y"=-8.599825, "Slope"=0.0}, {"X"=11.553976, "Y"=-8.164364, "Slope"=0.0}, {"X"=11.555473, "Y"=-8.257444, "Slope"=0.0}, {"X"=11.570158, "Y"=-8.345382, "Slope"=0.0}, {"X"=11.597317, "Y"=-8.425903, "Slope"=0.0}, {"X"=11.634399, "Y"=-8.4943, "Slope"=0.0}, {"X"=11.681087, "Y"=-8.552723, "Slope"=0.0}, {"X"=11.38384, "Y"=-13.431717, "Slope"=0.0}, {"X"=11.376223, "Y"=-13.986052, "Slope"=0.0}, {"X"=11.32265, "Y"=-14.114156, "Slope"=0.0}, {"X"=10.962178, "Y"=-14.504524, "Slope"=0.0}, {"X"=11.068745, "Y"=-14.428592, "Slope"=0.0}, {"X"=11.166584, "Y"=-14.337027, "Slope"=0.0}, {"X"=11.142837, "Y"=-14.359256, "Slope"=0.0}, {"X"=10.852696, "Y"=-14.562547, "Slope"=0.0}, {"X"=10.906145, "Y"=-14.535062, "Slope"=0.0}, {"X"=10.917822, "Y"=-12.891214, "Slope"=0.0}, {"X"=10.941155, "Y"=-12.903137, "Slope"=0.0}, {"X"=11.053217, "Y"=-12.9728775, "Slope"=0.0}, {"X"=11.152857, "Y"=-13.057631, "Slope"=0.0}, {"X"=11.241991, "Y"=-13.15944, "Slope"=0.0}, {"X"=11.318304, "Y"=-13.278711, "Slope"=0.0}, {"X"=11.3744755, "Y"=-13.408314, "Slope"=0.0}, {"X"=11.331289, "Y"=-13.300342, "Slope"=0.0}, {"X"=10.960146, "Y"=-12.914559, "Slope"=0.0}, {"X"=11.414788, "Y"=-13.569632, "Slope"=0.0}, {"X"=11.152857, "Y"=-13.057631, "Slope"=0.0}, {"X"=11.241991, "Y"=-13.15944, "Slope"=0.0}, {"X"=11.258465, "Y"=-13.179006, "Slope"=0.0}, {"X"=11.414788, "Y"=-13.569632, "Slope"=0.0}, {"X"=11.42357, "Y"=-13.710416, "Slope"=0.0}, {"X"=11.42357, "Y"=-13.710416, "Slope"=0.0}, {"X"=11.410399, "Y"=-13.850409, "Slope"=0.0}, {"X"=11.410399, "Y"=-13.850409, "Slope"=0.0}, {"X"=11.376223, "Y"=-13.986052, "Slope"=0.0}, {"X"=11.32265, "Y"=-14.114156, "Slope"=0.0}, {"X"=11.251816, "Y"=-14.232005, "Slope"=0.0}, {"X"=11.251816, "Y"=-14.232005, "Slope"=0.0}, {"X"=11.068745, "Y"=-14.428592, "Slope"=0.0}, {"X"=10.962178, "Y"=-14.504524, "Slope"=0.0}, {"X"=12.108151, "Y"=-5.9460087, "Slope"=0.0}, {"X"=11.915035, "Y"=-6.6864777, "Slope"=0.0}, {"X"=12.631411, "Y"=-4.049288, "Slope"=0.0}, {"X"=12.463001, "Y"=-4.6658015, "Slope"=0.0}, {"X"=12.140221, "Y"=-5.825948, "Slope"=0.0}, {"X"=12.201659, "Y"=-5.5894847, "Slope"=0.0}, {"X"=11.571496, "Y"=-8.037169, "Slope"=0.0}, {"X"=11.915035, "Y"=-6.6864777, "Slope"=0.0}, {"X"=10.66729, "Y"=-12.416573, "Slope"=0.0}, {"X"=10.664678, "Y"=-12.487158, "Slope"=0.0}, {"X"=10.664678, "Y"=-12.487158, "Slope"=0.0}, {"X"=10.670587, "Y"=-12.561274, "Slope"=0.0}, {"X"=10.688572, "Y"=-12.633139, "Slope"=0.0}, {"X"=10.718177, "Y"=-12.700924, "Slope"=0.0}, {"X"=10.755885, "Y"=-12.759442, "Slope"=0.0}, {"X"=10.802387, "Y"=-12.811512, "Slope"=0.0}, {"X"=10.85663, "Y"=-12.855927, "Slope"=0.0}, {"X"=10.665664, "Y"=-12.508651, "Slope"=0.0}, {"X"=10.675016, "Y"=-12.582449, "Slope"=0.0}, {"X"=10.696369, "Y"=-12.653376, "Slope"=0.0}, {"X"=10.729141, "Y"=-12.7196455, "Slope"=0.0}, {"X"=10.769699, "Y"=-12.776132, "Slope"=0.0}, {"X"=10.917822, "Y"=-12.891214, "Slope"=0.0}, {"X"=10.85663, "Y"=-12.855927, "Slope"=0.0}, {"X"=9.587701, "Y"=-14.956815, "Slope"=0.0}, {"X"=9.648387, "Y"=-14.928349, "Slope"=0.0}, {"X"=9.685769, "Y"=-14.907634, "Slope"=0.0}, {"X"=9.685769, "Y"=-14.907634, "Slope"=0.0}, {"X"=9.706607, "Y"=-14.895271, "Slope"=0.0}, {"X"=9.706607, "Y"=-14.895271, "Slope"=0.0}, {"X"=9.7413225, "Y"=-14.872915, "Slope"=0.0}, {"X"=9.773887, "Y"=-14.849932, "Slope"=0.0}, {"X"=9.789424, "Y"=-14.838251, "Slope"=0.0}, {"X"=9.789424, "Y"=-14.838251, "Slope"=0.0}, {"X"=9.8475485, "Y"=-14.790401, "Slope"=0.0}, {"X"=9.855697, "Y"=-14.783052, "Slope"=0.0}, {"X"=12.5287, "Y"=-3.5463154, "Slope"=0.0}, {"X"=12.579146, "Y"=-3.6137137, "Slope"=0.0}, {"X"=12.590708, "Y"=-3.6321623, "Slope"=0.0}, {"X"=12.590708, "Y"=-3.6321623, "Slope"=0.0}, {"X"=12.3426285, "Y"=-3.4355154, "Slope"=0.0}, {"X"=12.359256, "Y"=-3.4377937, "Slope"=0.0}, {"X"=12.359256, "Y"=-3.4377937, "Slope"=0.0}, {"X"=12.450331, "Y"=-3.4807534, "Slope"=0.0}, {"X"=12.450331, "Y"=-3.4807534, "Slope"=0.0}, {"X"=12.632841, "Y"=-3.7352073, "Slope"=0.0}, {"X"=12.632841, "Y"=-3.7352073, "Slope"=0.0}, {"X"=12.651887, "Y"=-3.8513145, "Slope"=0.0}, {"X"=12.651887, "Y"=-3.8513145, "Slope"=0.0}, {"X"=12.645298, "Y"=-3.9750311, "Slope"=0.0}, {"X"=12.645298, "Y"=-3.9750311, "Slope"=0.0}, {"X"=3.0186722, "Y"=-0.7281756, "Slope"=0.0}, {"X"=2.9258673, "Y"=-0.58080864, "Slope"=0.0}, {"X"=3.2307372, "Y"=-0.992266, "Slope"=0.0}, {"X"=3.0871935, "Y"=-0.82208127, "Slope"=0.0}, {"X"=3.1662605, "Y"=-0.9221965, "Slope"=0.0}, {"X"=3.4415681, "Y"=-1.1873536, "Slope"=0.0}, {"X"=3.355999, "Y"=-1.112888, "Slope"=0.0}, {"X"=3.2307372, "Y"=-0.992266, "Slope"=0.0}, {"X"=10.293746, "Y"=-14.642103, "Slope"=0.0}, {"X"=10.043219, "Y"=-14.665805, "Slope"=0.0}, {"X"=10.042806, "Y"=-14.666001, "Slope"=0.0}, {"X"=10.026867, "Y"=-14.673826, "Slope"=0.0}, {"X"=10.168064, "Y"=-14.638672, "Slope"=0.0}, {"X"=10.166119, "Y"=-14.639059, "Slope"=0.0}, {"X"=10.170087, "Y"=-14.63848, "Slope"=0.0}, {"X"=10.170087, "Y"=-14.63848, "Slope"=0.0}, {"X"=9.889225, "Y"=-14.7537775, "Slope"=0.0}, {"X"=9.886506, "Y"=-14.755914, "Slope"=0.0}, {"X"=9.861074, "Y"=-14.778302, "Slope"=0.0}, {"X"=9.861074, "Y"=-14.778302, "Slope"=0.0}, {"X"=9.566524, "Y"=-14.966767, "Slope"=0.0}, {"X"=9.549708, "Y"=-14.973137, "Slope"=0.0}, {"X"=9.417389, "Y"=-15.04401, "Slope"=0.0}, {"X"=9.439605, "Y"=-15.031419, "Slope"=0.0}, {"X"=9.494886, "Y"=-15.000398, "Slope"=0.0}, {"X"=9.531347, "Y"=-14.98244, "Slope"=0.0}, {"X"=9.507523, "Y"=-14.993372, "Slope"=0.0}, {"X"=9.462498, "Y"=-15.017409, "Slope"=0.0}, {"X"=4.7655854, "Y"=0.60666454, "Slope"=0.0}, {"X"=4.900757, "Y"=2.44138, "Slope"=0.0}, {"X"=4.445768, "Y"=2.35025, "Slope"=0.0}, {"X"=4.0750275, "Y"=2.213103, "Slope"=0.0}, {"X"=4.084907, "Y"=0.7651222, "Slope"=0.0}, {"X"=5.326706, "Y"=0.63066685, "Slope"=0.0}, {"X"=5.719236, "Y"=0.7264725, "Slope"=0.0}, {"X"=5.5209336, "Y"=2.4304006, "Slope"=0.0}, {"X"=3.8698528, "Y"=2.0458076, "Slope"=0.0}, {"X"=3.6970007, "Y"=1.864326, "Slope"=0.0}, {"X"=3.6070752, "Y"=1.2053412, "Slope"=0.0}, {"X"=3.7241516, "Y"=1.0319262, "Slope"=0.0}, {"X"=3.5714078, "Y"=1.6560217, "Slope"=0.0}, {"X"=3.5652642, "Y"=1.6428374, "Slope"=0.0}, {"X"=3.5714078, "Y"=1.6560217, "Slope"=0.0}, {"X"=3.5508623, "Y"=1.3571573, "Slope"=0.0}, {"X"=3.553045, "Y"=1.3868557, "Slope"=0.0}, {"X"=6.3881073, "Y"=1.1548297, "Slope"=0.0}, {"X"=6.4852514, "Y"=1.3510339, "Slope"=0.0}, {"X"=6.5348525, "Y"=1.5920166, "Slope"=0.0}, {"X"=6.4325643, "Y"=1.9461969, "Slope"=0.0}, {"X"=6.002293, "Y"=0.86890256, "Slope"=0.0}, {"X"=6.2358575, "Y"=1.0170529, "Slope"=0.0}, {"X"=6.320571, "Y"=2.0987613, "Slope"=0.0}, {"X"=5.2293944, "Y"=0.60893834, "Slope"=0.0}, {"X"=4.659784, "Y"=0.60572743, "Slope"=0.0}, {"X"=4.659784, "Y"=0.60572743, "Slope"=0.0}, {"X"=5.7946186, "Y"=0.74757576, "Slope"=0.0}, {"X"=5.5763397, "Y"=0.685647, "Slope"=0.0}, {"X"=4.084907, "Y"=0.7651222, "Slope"=0.0}, {"X"=6.352519, "Y"=1.1123196, "Slope"=0.0}, {"X"=6.1843343, "Y"=0.97466177, "Slope"=0.0}, {"X"=3.7241516, "Y"=1.0319262, "Slope"=0.0}, {"X"=6.4053516, "Y"=1.1754698, "Slope"=0.0}, {"X"=6.5370927, "Y"=1.4654024, "Slope"=0.0}, {"X"=6.531951, "Y"=1.7503738, "Slope"=0.0}, {"X"=3.6970007, "Y"=1.864326, "Slope"=0.0}, {"X"=3.8698528, "Y"=2.0458076, "Slope"=0.0}, {"X"=4.1120195, "Y"=2.2329714, "Slope"=0.0}, {"X"=6.3898935, "Y"=2.0303822, "Slope"=0.0}, {"X"=5.740962, "Y"=2.4042594, "Slope"=0.0}, {"X"=5.1689224, "Y"=2.4760795, "Slope"=0.0}, {"X"=4.445768, "Y"=2.35025, "Slope"=0.0}, {"X"=4.6014295, "Y"=2.4074922, "Slope"=0.0}, {"X"=4.8172107, "Y"=7.1894627, "Slope"=0.0}, {"X"=5.491926, "Y"=7.8015456, "Slope"=0.0}, {"X"=5.7070355, "Y"=7.828284, "Slope"=0.0}, {"X"=5.966891, "Y"=7.8276443, "Slope"=0.0}, {"X"=6.2695904, "Y"=7.7851615, "Slope"=0.0}, {"X"=6.6780767, "Y"=7.650669, "Slope"=0.0}, {"X"=6.705697, "Y"=7.639021, "Slope"=0.0}, {"X"=5.022007, "Y"=7.5899568, "Slope"=0.0}, {"X"=4.9459004, "Y"=7.5142617, "Slope"=0.0}, {"X"=4.884291, "Y"=7.4300137, "Slope"=0.0}, {"X"=4.8388834, "Y"=7.3348093, "Slope"=0.0}, {"X"=4.8172107, "Y"=7.1894627, "Slope"=0.0}, {"X"=5.3497233, "Y"=7.7608624, "Slope"=0.0}, {"X"=5.2258754, "Y"=7.7112513, "Slope"=0.0}, {"X"=5.113709, "Y"=7.657008, "Slope"=0.0}, {"X"=5.7070355, "Y"=7.828284, "Slope"=0.0}, {"X"=5.966891, "Y"=7.8276443, "Slope"=0.0}, {"X"=6.2695904, "Y"=7.7851615, "Slope"=0.0}, {"X"=5.022007, "Y"=7.5899568, "Slope"=0.0}, {"X"=5.121181, "Y"=7.66165, "Slope"=0.0}, {"X"=5.0031524, "Y"=7.5747905, "Slope"=0.0}, {"X"=5.2258754, "Y"=7.7112513, "Slope"=0.0}, {"X"=4.8388834, "Y"=7.3348093, "Slope"=0.0}, {"X"=4.884291, "Y"=7.4300137, "Slope"=0.0}, {"X"=5.491926, "Y"=7.8015456, "Slope"=0.0}, {"X"=5.4493246, "Y"=7.7930207, "Slope"=0.0}, {"X"=6.835574, "Y"=7.554695, "Slope"=0.0}, {"X"=6.8738914, "Y"=7.5214505, "Slope"=0.0}, {"X"=6.824801, "Y"=7.5637803, "Slope"=0.0}, {"X"=6.705697, "Y"=7.639021, "Slope"=0.0}, {"X"=6.710484, "Y"=7.6377482, "Slope"=0.0}, {"X"=6.79099, "Y"=7.591445, "Slope"=0.0}, {"X"=6.779359, "Y"=7.5995193, "Slope"=0.0}, {"X"=6.895845, "Y"=7.488816, "Slope"=0.0}, {"X"=6.8901258, "Y"=7.503174, "Slope"=0.0}, {"X"=6.8738914, "Y"=7.5214505, "Slope"=0.0}, {"X"=6.8476286, "Y"=7.5443726, "Slope"=0.0}, {"X"=6.8445525, "Y"=7.5470734, "Slope"=0.0}, {"X"=6.79099, "Y"=7.591445, "Slope"=0.0}, {"X"=6.824801, "Y"=7.5637803, "Slope"=0.0}, {"X"=6.835574, "Y"=7.554695, "Slope"=0.0}, {"X"=6.871907, "Y"=7.523237, "Slope"=0.0}, {"X"=6.864228, "Y"=7.5299687, "Slope"=0.0}, {"X"=7.067577, "Y"=7.3290687, "Slope"=0.0}, {"X"=7.0931997, "Y"=7.302365, "Slope"=0.0}, {"X"=7.006349, "Y"=6.472289, "Slope"=0.0}, {"X"=7.0611887, "Y"=6.5513105, "Slope"=0.0}, {"X"=7.1854534, "Y"=6.8420715, "Slope"=0.0}, {"X"=7.2024646, "Y"=7.019425, "Slope"=0.0}, {"X"=7.067577, "Y"=7.3290687, "Slope"=0.0}, {"X"=7.0931997, "Y"=7.302365, "Slope"=0.0}, {"X"=7.175538, "Y"=6.74118, "Slope"=0.0}, {"X"=9.953516, "Y"=-14.708637, "Slope"=0.0}, {"X"=10.026867, "Y"=-14.673826, "Slope"=0.0}, {"X"=9.903194, "Y"=-14.742871, "Slope"=0.0}, {"X"=9.417389, "Y"=-15.04401, "Slope"=0.0}, {"X"=9.369135, "Y"=-15.07428, "Slope"=0.0}, {"X"=8.505421, "Y"=-15.596214, "Slope"=0.0}, {"X"=8.491675, "Y"=-15.604596, "Slope"=0.0}, {"X"=9.267097, "Y"=-15.138879, "Slope"=0.0}, {"X"=9.267097, "Y"=-15.138879, "Slope"=0.0}, {"X"=8.937251, "Y"=-15.3406515, "Slope"=0.0}, {"X"=8.282294, "Y"=-15.731429, "Slope"=0.0}, {"X"=8.050529, "Y"=-15.86282, "Slope"=0.0}, {"X"=8.069378, "Y"=-15.8505335, "Slope"=0.0}, {"X"=7.6827683, "Y"=-16.072777, "Slope"=0.0}, {"X"=7.5478926, "Y"=-16.157545, "Slope"=0.0}, {"X"=9.187492, "Y"=-15.184627, "Slope"=0.0}, {"X"=8.862729, "Y"=-15.382493, "Slope"=0.0}, {"X"=8.282294, "Y"=-15.731429, "Slope"=0.0}, {"X"=8.4929, "Y"=-15.603772, "Slope"=0.0}, {"X"=7.430489, "Y"=-16.223211, "Slope"=0.0}, {"X"=7.5478926, "Y"=-16.157545, "Slope"=0.0}, {"X"=7.171605, "Y"=-16.371065, "Slope"=0.0}, {"X"=7.171605, "Y"=-16.371065, "Slope"=0.0}, {"X"=11.320335, "Y"=-10.768083, "Slope"=0.0}, {"X"=11.929371, "Y"=-10.2494545, "Slope"=0.0}, {"X"=11.917312, "Y"=-10.265866, "Slope"=0.0}, {"X"=11.885427, "Y"=-10.314343, "Slope"=0.0}, {"X"=11.885427, "Y"=-10.314343, "Slope"=0.0}, {"X"=11.834314, "Y"=-10.379304, "Slope"=0.0}, {"X"=11.74231, "Y"=-10.482889, "Slope"=0.0}, {"X"=11.640282, "Y"=-10.577035, "Slope"=0.0}, {"X"=11.544385, "Y"=-10.650674, "Slope"=0.0}, {"X"=11.86617, "Y"=-10.3413925, "Slope"=0.0}, {"X"=11.295982, "Y"=-10.777359, "Slope"=0.0}, {"X"=11.312095, "Y"=-10.770921, "Slope"=0.0}, {"X"=11.640282, "Y"=-10.577035, "Slope"=0.0}, {"X"=11.74231, "Y"=-10.482889, "Slope"=0.0}, {"X"=11.282086, "Y"=-10.783227, "Slope"=0.0}, {"X"=11.213371, "Y"=-10.816897, "Slope"=0.0}, {"X"=11.14764, "Y"=-10.85966, "Slope"=0.0}, {"X"=11.086128, "Y"=-10.911853, "Slope"=0.0}, {"X"=11.295982, "Y"=-10.777359, "Slope"=0.0}, {"X"=11.029917, "Y"=-10.97244, "Slope"=0.0}, {"X"=10.975225, "Y"=-11.048819, "Slope"=0.0}, {"X"=10.929667, "Y"=-11.131481, "Slope"=0.0}, {"X"=10.894082, "Y"=-11.2184515, "Slope"=0.0}, {"X"=10.870948, "Y"=-11.297758, "Slope"=0.0}, {"X"=10.887574, "Y"=-11.235525, "Slope"=0.0}, {"X"=11.029917, "Y"=-10.97244, "Slope"=0.0}, {"X"=11.0298, "Y"=-10.972571, "Slope"=0.0}, {"X"=10.971792, "Y"=-11.053841, "Slope"=0.0}, {"X"=10.924006, "Y"=-11.142319, "Slope"=0.0}, {"X"=11.086128, "Y"=-10.911853, "Slope"=0.0}, {"X"=11.14764, "Y"=-10.85966, "Slope"=0.0}, {"X"=11.213371, "Y"=-10.816897, "Slope"=0.0}, {"X"=10.301758, "Y"=-14.642538, "Slope"=0.0}, {"X"=10.293746, "Y"=-14.642103, "Slope"=0.0}, {"X"=10.564897, "Y"=-14.646091, "Slope"=0.0}, {"X"=10.851432, "Y"=-14.563225, "Slope"=0.0}, {"X"=10.747182, "Y"=-14.602583, "Slope"=0.0}, {"X"=10.712086, "Y"=-14.615379, "Slope"=0.0}, {"X"=10.564897, "Y"=-14.646091, "Slope"=0.0}, {"X"=10.862119, "Y"=-11.333081, "Slope"=0.0}, {"X"=10.7726345, "Y"=-11.824437, "Slope"=0.0}, {"X"=10.677209, "Y"=-12.364202, "Slope"=0.0}, {"X"=10.66729, "Y"=-12.416573, "Slope"=0.0}, {"X"=4.963912, "Y"=6.637194, "Slope"=0.0}, {"X"=4.8515596, "Y"=6.9179187, "Slope"=0.0}, {"X"=4.8176155, "Y"=7.048952, "Slope"=0.0}, {"X"=5.0467963, "Y"=6.464496, "Slope"=0.0}, {"X"=5.8659306, "Y"=5.9515653, "Slope"=0.0}, {"X"=5.8659306, "Y"=5.9515653, "Slope"=0.0}, {"X"=5.9262633, "Y"=5.951276, "Slope"=0.0}, {"X"=6.33229, "Y"=6.0232587, "Slope"=0.0}, {"X"=6.33229, "Y"=6.0232587, "Slope"=0.0}, {"X"=6.629424, "Y"=6.1670747, "Slope"=0.0}, {"X"=6.629424, "Y"=6.1670747, "Slope"=0.0}, {"X"=6.817724, "Y"=6.3108954, "Slope"=0.0}, {"X"=7.006349, "Y"=6.472289, "Slope"=0.0}, {"X"=5.0467963, "Y"=6.464496, "Slope"=0.0}, {"X"=5.164426, "Y"=6.294174, "Slope"=0.0}, {"X"=5.293289, "Y"=6.1826806, "Slope"=0.0}, {"X"=5.4052844, "Y"=6.1176023, "Slope"=0.0}, {"X"=5.54563, "Y"=6.0281105, "Slope"=0.0}, {"X"=5.54563, "Y"=6.0281105, "Slope"=0.0}, {"X"=5.5747533, "Y"=6.0193143, "Slope"=0.0}, {"X"=-4.928284, "Y"=-17.347603, "Slope"=0.0}, {"X"=-4.485192, "Y"=-17.473867, "Slope"=0.0}, {"X"=-4.0872045, "Y"=-17.574154, "Slope"=0.0}, {"X"=-6.636535, "Y"=-16.656498, "Slope"=0.0}, {"X"=-6.955111, "Y"=-16.489447, "Slope"=0.0}, {"X"=-7.032068, "Y"=-16.445217, "Slope"=0.0}, {"X"=-6.440816, "Y"=-16.758366, "Slope"=0.0}, {"X"=-6.1145263, "Y"=-16.906958, "Slope"=0.0}, {"X"=-6.048642, "Y"=-16.935936, "Slope"=0.0}, {"X"=-5.657333, "Y"=-17.094572, "Slope"=0.0}, {"X"=-4.8739295, "Y"=-17.364567, "Slope"=0.0}, {"X"=-3.6903965, "Y"=-17.662962, "Slope"=0.0}, {"X"=-3.2915175, "Y"=-17.736147, "Slope"=0.0}, {"X"=-5.265338, "Y"=-17.239439, "Slope"=0.0}, {"X"=-6.636535, "Y"=-16.656498, "Slope"=0.0}, {"X"=-6.1145263, "Y"=-16.906958, "Slope"=0.0}, {"X"=-6.3764787, "Y"=-16.788654, "Slope"=0.0}, {"X"=-5.657333, "Y"=-17.094572, "Slope"=0.0}, {"X"=-5.531905, "Y"=-17.140982, "Slope"=0.0}, {"X"=-5.2347617, "Y"=-17.249676, "Slope"=0.0}, {"X"=-4.8739295, "Y"=-17.364567, "Slope"=0.0}, {"X"=-4.485192, "Y"=-17.473867, "Slope"=0.0}, {"X"=-4.0872045, "Y"=-17.574154, "Slope"=0.0}, {"X"=-3.6903965, "Y"=-17.662962, "Slope"=0.0}, {"X"=3.6075315, "Y"=-17.680258, "Slope"=0.0}, {"X"=6.638166, "Y"=-16.656498, "Slope"=0.0}, {"X"=6.781946, "Y"=-16.580774, "Slope"=0.0}, {"X"=6.956742, "Y"=-16.489447, "Slope"=0.0}, {"X"=6.781946, "Y"=-16.580774, "Slope"=0.0}, {"X"=3.6075315, "Y"=-17.680258, "Slope"=0.0}, {"X"=3.7670631, "Y"=-17.646334, "Slope"=0.0}, {"X"=6.2929645, "Y"=-16.828487, "Slope"=0.0}, {"X"=5.9106174, "Y"=-16.992453, "Slope"=0.0}, {"X"=5.3245015, "Y"=-17.21816, "Slope"=0.0}, {"X"=5.133149, "Y"=-17.284317, "Slope"=0.0}, {"X"=4.7839193, "Y"=-17.390415, "Slope"=0.0}, {"X"=3.6920273, "Y"=-17.662962, "Slope"=0.0}, {"X"=6.2929645, "Y"=-16.828487, "Slope"=0.0}, {"X"=6.050273, "Y"=-16.935936, "Slope"=0.0}, {"X"=5.6589637, "Y"=-17.094572, "Slope"=0.0}, {"X"=5.2669687, "Y"=-17.239439, "Slope"=0.0}, {"X"=4.8755603, "Y"=-17.364567, "Slope"=0.0}, {"X"=4.4868226, "Y"=-17.473867, "Slope"=0.0}, {"X"=4.298019, "Y"=-17.521143, "Slope"=0.0}, {"X"=-10.260574, "Y"=-3.3069108, "Slope"=0.0}, {"X"=-11.283855, "Y"=-3.3711903, "Slope"=0.0}, {"X"=-9.970092, "Y"=-3.2923765, "Slope"=0.0}, {"X"=-3.4399374, "Y"=-1.1873536, "Slope"=0.0}, {"X"=-3.521916, "Y"=-1.2533891, "Slope"=0.0}, {"X"=-3.7573729, "Y"=-1.434901, "Slope"=0.0}, {"X"=-3.7573729, "Y"=-1.434901, "Slope"=0.0}, {"X"=-4.0478854, "Y"=-1.6355752, "Slope"=0.0}, {"X"=-4.3772445, "Y"=-1.8462685, "Slope"=0.0}, {"X"=-5.34146, "Y"=-2.3618393, "Slope"=0.0}, {"X"=-5.662619, "Y"=-2.4989357, "Slope"=0.0}, {"X"=-5.024132, "Y"=-2.209944, "Slope"=0.0}, {"X"=-4.7063894, "Y"=-2.058018, "Slope"=0.0}, {"X"=-4.711721, "Y"=-2.061136, "Slope"=0.0}, {"X"=-6.1184225, "Y"=-2.6457238, "Slope"=0.0}, {"X"=-6.607805, "Y"=-2.8040211, "Slope"=0.0}, {"X"=-12.232183, "Y"=-3.4180868, "Slope"=0.0}, {"X"=-12.128426, "Y"=-3.4163973, "Slope"=0.0}, {"X"=-12.232183, "Y"=-3.4180868, "Slope"=0.0}, {"X"=-8.707709, "Y"=-3.1807067, "Slope"=0.0}, {"X"=-9.8188925, "Y"=-3.2787843, "Slope"=0.0}, {"X"=-9.738416, "Y"=-3.2713087, "Slope"=0.0}, {"X"=-9.06884, "Y"=-3.2148187, "Slope"=0.0}, {"X"=-8.707709, "Y"=-3.1807067, "Slope"=0.0}, {"X"=-7.530573, "Y"=-3.0147233, "Slope"=0.0}, {"X"=-11.738921, "Y"=-3.3929737, "Slope"=0.0}, {"X"=-11.843679, "Y"=-3.4006338, "Slope"=0.0}, {"X"=-11.843679, "Y"=-3.4006338, "Slope"=0.0}, {"X"=-10.702967, "Y"=-3.3331478, "Slope"=0.0}, {"X"=-11.072473, "Y"=-3.354675, "Slope"=0.0}, {"X"=-11.1448, "Y"=-3.3608747, "Slope"=0.0}, {"X"=-10.260574, "Y"=-3.3069108, "Slope"=0.0}, {"X"=-11.283855, "Y"=-3.3711903, "Slope"=0.0}, {"X"=-9.380922, "Y"=-3.240731, "Slope"=0.0}, {"X"=-6.607805, "Y"=-2.8040211, "Slope"=0.0}, {"X"=-8.248184, "Y"=-3.1152034, "Slope"=0.0}, {"X"=-7.7203517, "Y"=-3.047589, "Slope"=0.0}, {"X"=-7.119101, "Y"=-2.9200442, "Slope"=0.0}, {"X"=-5.662619, "Y"=-2.4989357, "Slope"=0.0}, {"X"=-6.1184225, "Y"=-2.6457238, "Slope"=0.0}, {"X"=-5.34146, "Y"=-2.3618393, "Slope"=0.0}, {"X"=-5.221523, "Y"=-2.3109796, "Slope"=0.0}, {"X"=-4.0478854, "Y"=-1.6355752, "Slope"=0.0}, {"X"=-4.3772445, "Y"=-1.8462685, "Slope"=0.0}, {"X"=12.233814, "Y"=-3.4180868, "Slope"=0.0}, {"X"=12.130056, "Y"=-3.4163973, "Slope"=0.0}, {"X"=11.893608, "Y"=-3.404276, "Slope"=0.0}, {"X"=11.84531, "Y"=-3.4006338, "Slope"=0.0}, {"X"=9.479367, "Y"=-3.2494392, "Slope"=0.0}, {"X"=11.740552, "Y"=-3.3929737, "Slope"=0.0}, {"X"=7.7219825, "Y"=-3.047589, "Slope"=0.0}, {"X"=5.7348065, "Y"=-2.5273833, "Slope"=0.0}, {"X"=4.692581, "Y"=-2.0487688, "Slope"=0.0}, {"X"=5.2231536, "Y"=-2.3109796, "Slope"=0.0}, {"X"=4.7049255, "Y"=-2.056361, "Slope"=0.0}, {"X"=4.692581, "Y"=-2.0487688, "Slope"=0.0}, {"X"=3.7590036, "Y"=-1.434901, "Slope"=0.0}, {"X"=3.6075091, "Y"=-1.3226423, "Slope"=0.0}, {"X"=3.6075091, "Y"=-1.3226423, "Slope"=0.0}, {"X"=3.4415681, "Y"=-1.1873536, "Slope"=0.0}, {"X"=5.7348065, "Y"=-2.5273833, "Slope"=0.0}, {"X"=10.849632, "Y"=-3.3406618, "Slope"=0.0}, {"X"=11.84531, "Y"=-3.4006338, "Slope"=0.0}, {"X"=11.285486, "Y"=-3.3711903, "Slope"=0.0}, {"X"=10.407241, "Y"=-3.3139515, "Slope"=0.0}, {"X"=9.7400465, "Y"=-3.2713087, "Slope"=0.0}, {"X"=9.479367, "Y"=-3.2494392, "Slope"=0.0}, {"X"=10.407241, "Y"=-3.3139515, "Slope"=0.0}, {"X"=8.70934, "Y"=-3.1807067, "Slope"=0.0}, {"X"=7.7219825, "Y"=-3.047589, "Slope"=0.0}, {"X"=7.5322037, "Y"=-3.0147233, "Slope"=0.0}, {"X"=6.7377086, "Y"=-2.841617, "Slope"=0.0}, {"X"=5.2231536, "Y"=-2.3109796, "Slope"=0.0}, {"X"=4.173215, "Y"=-1.7233979, "Slope"=0.0}, {"X"=2.092016, "Y"=-17.90657, "Slope"=0.0}, {"X"=0.42150292, "Y"=-18.00863, "Slope"=0.0}, {"X"=0.34319338, "Y"=-18.009645, "Slope"=0.0}, {"X"=1.695347, "Y"=-17.944841, "Slope"=0.0}, {"X"=3.1908336, "Y"=-17.753933, "Slope"=0.0}, {"X"=2.9825726, "Y"=-17.7882, "Slope"=0.0}, {"X"=2.7701542, "Y"=-17.82051, "Slope"=0.0}, {"X"=2.5594132, "Y"=-17.850025, "Slope"=0.0}, {"X"=2.490218, "Y"=-17.859251, "Slope"=0.0}, {"X"=3.2931483, "Y"=-17.736147, "Slope"=0.0}, {"X"=2.0012887, "Y"=-17.915014, "Slope"=0.0}, {"X"=2.0012887, "Y"=-17.915014, "Slope"=0.0}, {"X"=0.84556794, "Y"=-17.997324, "Slope"=0.0}, {"X"=0.44709656, "Y"=-18.008022, "Slope"=0.0}, {"X"=0.42150292, "Y"=-18.00863, "Slope"=0.0}, {"X"=1.3231481, "Y"=-17.972385, "Slope"=0.0}, {"X"=1.2700415, "Y"=-17.976114, "Slope"=0.0}, {"X"=2.690039, "Y"=-17.832129, "Slope"=0.0}, {"X"=2.7701542, "Y"=-17.82051, "Slope"=0.0}, {"X"=3.0914207, "Y"=-17.77078, "Slope"=0.0}, {"X"=0.0008154644, "Y"=-18.009115, "Slope"=0.0}, {"X"=-0.0014298288, "Y"=-18.008503, "Slope"=0.0}, {"X"=0.0037170372, "Y"=-18.006178, "Slope"=0.0}, {"X"=0.0030606594, "Y"=-18.008503, "Slope"=0.0}, {"X"=-2.0903852, "Y"=-17.90657, "Slope"=0.0}, {"X"=-3.2915175, "Y"=-17.736147, "Slope"=0.0}, {"X"=-3.1892028, "Y"=-17.753933, "Slope"=0.0}, {"X"=-2.9965718, "Y"=-17.78538, "Slope"=0.0}, {"X"=-2.8064823, "Y"=-17.814571, "Slope"=0.0}, {"X"=-2.616186, "Y"=-17.841745, "Slope"=0.0}, {"X"=-2.3674042, "Y"=-17.87328, "Slope"=0.0}, {"X"=-2.4885871, "Y"=-17.859251, "Slope"=0.0}, {"X"=-0.0020862846, "Y"=-18.006178, "Slope"=0.0}, {"X"=-0.07978936, "Y"=-18.006723, "Slope"=0.0}, {"X"=-0.34159136, "Y"=-18.009645, "Slope"=0.0}, {"X"=-0.8106943, "Y"=-17.998108, "Slope"=0.0}, {"X"=-1.2199664, "Y"=-17.978369, "Slope"=0.0}, {"X"=-1.6231827, "Y"=-17.949776, "Slope"=0.0}, {"X"=-1.6937162, "Y"=-17.944841, "Slope"=0.0}, {"X"=-1.6231827, "Y"=-17.949776, "Slope"=0.0}, {"X"=-2.616186, "Y"=-17.841745, "Slope"=0.0}, {"X"=-2.8064823, "Y"=-17.814571, "Slope"=0.0}, {"X"=-3.0897899, "Y"=-17.77078, "Slope"=0.0}, {"X"=-1.2199664, "Y"=-17.978369, "Slope"=0.0}, {"X"=-0.8106943, "Y"=-17.998108, "Slope"=0.0}, {"X"=-0.00854867, "Y"=3.7263947, "Slope"=0.0}, {"X"=-0.0066404296, "Y"=3.7263823, "Slope"=0.0}, {"X"=0.008271213, "Y"=3.7263823, "Slope"=0.0}, {"X"=-0.76231277, "Y"=2.8479533, "Slope"=0.0}, {"X"=0.6740086, "Y"=2.847094, "Slope"=0.0}, {"X"=0.6740086, "Y"=2.847094, "Slope"=0.0}, {"X"=0.47253898, "Y"=2.847094, "Slope"=0.0}, {"X"=-0.07608838, "Y"=3.7179072, "Slope"=0.0}, {"X"=-0.4628392, "Y"=3.5587547, "Slope"=0.0}, {"X"=-0.3386752, "Y"=3.6528666, "Slope"=0.0}, {"X"=-0.07608838, "Y"=3.7179072, "Slope"=0.0}, {"X"=0.29774323, "Y"=3.670729, "Slope"=0.0}, {"X"=0.34028584, "Y"=3.6528666, "Slope"=0.0}, {"X"=0.46445665, "Y"=3.5587547, "Slope"=0.0}, {"X"=0.060030755, "Y"=3.720132, "Slope"=0.0}, {"X"=0.0101794535, "Y"=3.7263947, "Slope"=0.0}, {"X"=-0.4628392, "Y"=3.5587547, "Slope"=0.0}, {"X"=-0.49247614, "Y"=3.5338767, "Slope"=0.0}, {"X"=-0.49247614, "Y"=3.5338767, "Slope"=0.0}, {"X"=-0.48612607, "Y"=3.5097697, "Slope"=0.0}, {"X"=-0.45324963, "Y"=3.4870713, "Slope"=0.0}, {"X"=-0.39212748, "Y"=3.466576, "Slope"=0.0}, {"X"=-0.49027306, "Y"=3.5230303, "Slope"=0.0}, {"X"=-0.47441077, "Y"=3.5007813, "Slope"=0.0}, {"X"=-0.4386713, "Y"=3.4815457, "Slope"=0.0}, {"X"=-0.3861084, "Y"=3.465226, "Slope"=0.0}, {"X"=-0.24353056, "Y"=3.4534297, "Slope"=0.0}, {"X"=-0.36558542, "Y"=3.4612727, "Slope"=0.0}, {"X"=0.010381071, "Y"=3.4437823, "Slope"=0.0}, {"X"=-0.008876924, "Y"=3.4437895, "Slope"=0.0}, {"X"=-0.008750289, "Y"=3.4437823, "Slope"=0.0}, {"X"=0.010381071, "Y"=3.4437823, "Slope"=0.0}, {"X"=0.48574132, "Y"=3.544352, "Slope"=0.0}, {"X"=0.46445665, "Y"=3.5587547, "Slope"=0.0}, {"X"=0.4877475, "Y"=3.5097704, "Slope"=0.0}, {"X"=0.49189267, "Y"=3.5230253, "Slope"=0.0}, {"X"=0.49409693, "Y"=3.5338771, "Slope"=0.0}, {"X"=0.45487154, "Y"=3.4870725, "Slope"=0.0}, {"X"=0.4760247, "Y"=3.5007768, "Slope"=0.0}, {"X"=0.39375165, "Y"=3.466578, "Slope"=0.0}, {"X"=0.44027802, "Y"=3.4815414, "Slope"=0.0}, {"X"=0.24528153, "Y"=3.4534278, "Slope"=0.0}, {"X"=0.38770628, "Y"=3.465222, "Slope"=0.0}, {"X"=0.0105077075, "Y"=3.4437895, "Slope"=0.0}, {"X"=1.067618, "Y"=2.7614944, "Slope"=0.0}, {"X"=1.0173168, "Y"=2.8046827, "Slope"=0.0}, {"X"=1.0106434, "Y"=2.8081396, "Slope"=0.0}, {"X"=0.998331, "Y"=2.8126178, "Slope"=0.0}, {"X"=0.96865463, "Y"=2.8240356, "Slope"=0.0}, {"X"=0.96865463, "Y"=2.8240356, "Slope"=0.0}, {"X"=1.0473349, "Y"=2.7850795, "Slope"=0.0}, {"X"=1.0565383, "Y"=2.7741954, "Slope"=0.0}, {"X"=0.92898184, "Y"=2.8333485, "Slope"=0.0}, {"X"=0.92898184, "Y"=2.8333485, "Slope"=0.0}, {"X"=0.8959438, "Y"=2.8382154, "Slope"=0.0}, {"X"=0.8375098, "Y"=2.8446708, "Slope"=0.0}, {"X"=0.88944787, "Y"=2.8387268, "Slope"=0.0}, {"X"=0.7639368, "Y"=2.8479538, "Slope"=0.0}, {"X"=-1.045704, "Y"=2.7850792, "Slope"=0.0}, {"X"=-1.0445257, "Y"=2.7859926, "Slope"=0.0}, {"X"=-1.045704, "Y"=2.7850792, "Slope"=0.0}, {"X"=-1.0090119, "Y"=2.8081396, "Slope"=0.0}, {"X"=-0.9670265, "Y"=2.8240356, "Slope"=0.0}, {"X"=-0.8358763, "Y"=2.8446715, "Slope"=0.0}, {"X"=-0.7951621, "Y"=2.8454816, "Slope"=0.0}, {"X"=-0.7951621, "Y"=2.8454816, "Slope"=0.0}, {"X"=-0.8943183, "Y"=2.8382156, "Slope"=0.0}, {"X"=-0.8982203, "Y"=2.8373964, "Slope"=0.0}, {"X"=-0.8982203, "Y"=2.8373964, "Slope"=0.0}, {"X"=-0.9967021, "Y"=2.812618, "Slope"=0.0}, {"X"=-1.0090119, "Y"=2.8081396, "Slope"=0.0}, {"X"=-1.0659869, "Y"=2.7614949, "Slope"=0.0}, {"X"=-1.0549076, "Y"=2.7741952, "Slope"=0.0}, {"X"=-0.48852873, "Y"=2.3884056, "Slope"=0.0}, {"X"=-0.07730713, "Y"=2.3884056, "Slope"=0.0}, {"X"=0.7514543, "Y"=2.386611, "Slope"=0.0}, {"X"=-0.07730713, "Y"=2.3884056, "Slope"=0.0}, {"X"=-1.14167, "Y"=2.3826506, "Slope"=0.0}, {"X"=1.1432979, "Y"=2.3826497, "Slope"=0.0}, {"X"=-0.41324222, "Y"=2.0111115, "Slope"=0.0}, {"X"=-0.70813435, "Y"=2.0103872, "Slope"=0.0}, {"X"=-0.49057758, "Y"=2.0111115, "Slope"=0.0}, {"X"=0.70983547, "Y"=2.0103867, "Slope"=0.0}, {"X"=0.70983547, "Y"=2.0103867, "Slope"=0.0}, {"X"=-0.41324222, "Y"=2.0111115, "Slope"=0.0}, {"X"=1.2337487, "Y"=2.4588747, "Slope"=0.0}, {"X"=1.2165025, "Y"=2.404758, "Slope"=0.0}, {"X"=1.1983142, "Y"=2.397272, "Slope"=0.0}, {"X"=1.1722122, "Y"=2.3927495, "Slope"=0.0}, {"X"=1.1916199, "Y"=2.3954153, "Slope"=0.0}, {"X"=1.1432979, "Y"=2.3826497, "Slope"=0.0}, {"X"=1.2353605, "Y"=2.4271605, "Slope"=0.0}, {"X"=1.228462, "Y"=2.4146354, "Slope"=0.0}, {"X"=1.222558, "Y"=2.4088516, "Slope"=0.0}, {"X"=1.2165025, "Y"=2.404758, "Slope"=0.0}, {"X"=1.226176, "Y"=2.4763017, "Slope"=0.0}, {"X"=1.2289872, "Y"=2.4697802, "Slope"=0.0}, {"X"=1.2092305, "Y"=2.4009252, "Slope"=0.0}, {"X"=1.2353605, "Y"=2.4271605, "Slope"=0.0}, {"X"=1.2364476, "Y"=2.433267, "Slope"=0.0}, {"X"=1.2370933, "Y"=2.441883, "Slope"=0.0}, {"X"=1.4738536, "Y"=2.006581, "Slope"=0.0}, {"X"=1.4669265, "Y"=2.0087044, "Slope"=0.0}, {"X"=1.4593807, "Y"=2.009836, "Slope"=0.0}, {"X"=1.4574188, "Y"=2.009671, "Slope"=0.0}, {"X"=1.5014237, "Y"=1.9812346, "Slope"=0.0}, {"X"=1.4986236, "Y"=1.9855362, "Slope"=0.0}, {"X"=1.4926502, "Y"=1.9933399, "Slope"=0.0}, {"X"=1.4872434, "Y"=1.9984872, "Slope"=0.0}, {"X"=1.4812546, "Y"=2.0027587, "Slope"=0.0}, {"X"=1.4748765, "Y"=2.0060189, "Slope"=0.0}, {"X"=1.4802402, "Y"=2.0035176, "Slope"=0.0}, {"X"=1.4971714, "Y"=1.9878777, "Slope"=0.0}, {"X"=1.4920352, "Y"=1.9941158, "Slope"=0.0}, {"X"=1.4863943, "Y"=1.9993223, "Slope"=0.0}, {"X"=1.4593807, "Y"=2.009836, "Slope"=0.0}, {"X"=1.459968, "Y"=2.0097, "Slope"=0.0}, {"X"=-1.4576082, "Y"=2.009493, "Slope"=0.0}, {"X"=-1.457856, "Y"=2.0095024, "Slope"=0.0}, {"X"=-1.457856, "Y"=2.0095024, "Slope"=0.0}, {"X"=-1.4649794, "Y"=2.008526, "Slope"=0.0}, {"X"=-1.4716955, "Y"=2.0065548, "Slope"=0.0}, {"X"=-1.4780617, "Y"=2.0036175, "Slope"=0.0}, {"X"=-1.4843178, "Y"=1.9994733, "Slope"=0.0}, {"X"=-1.4902166, "Y"=1.9941378, "Slope"=0.0}, {"X"=-1.4956957, "Y"=1.9875569, "Slope"=0.0}, {"X"=-1.4960741, "Y"=1.986977, "Slope"=0.0}, {"X"=-1.4960741, "Y"=1.986977, "Slope"=0.0}, {"X"=-1.4579788, "Y"=2.009514, "Slope"=0.0}, {"X"=-1.4956957, "Y"=1.9875569, "Slope"=0.0}, {"X"=-1.4902166, "Y"=1.9941378, "Slope"=0.0}, {"X"=-1.4843178, "Y"=1.9994733, "Slope"=0.0}, {"X"=-1.4780617, "Y"=2.0036175, "Slope"=0.0}, {"X"=-1.4716955, "Y"=2.0065548, "Slope"=0.0}, {"X"=-1.2316467, "Y"=2.459709, "Slope"=0.0}, {"X"=-1.1959518, "Y"=2.398109, "Slope"=0.0}, {"X"=-1.1960353, "Y"=2.3981266, "Slope"=0.0}, {"X"=-1.2158687, "Y"=2.406542, "Slope"=0.0}, {"X"=-1.2276436, "Y"=2.4172268, "Slope"=0.0}, {"X"=-1.2336802, "Y"=2.4300911, "Slope"=0.0}, {"X"=-1.2346641, "Y"=2.4445548, "Slope"=0.0}, {"X"=-1.2352839, "Y"=2.442157, "Slope"=0.0}, {"X"=-1.1959518, "Y"=2.398109, "Slope"=0.0}, {"X"=-1.1648246, "Y"=2.3918023, "Slope"=0.0}, {"X"=-1.1706961, "Y"=2.3924835, "Slope"=0.0}, {"X"=-1.2245513, "Y"=2.476303, "Slope"=0.0}, {"X"=-1.2336527, "Y"=2.4271784, "Slope"=0.0}, {"X"=-1.2276436, "Y"=2.4172268, "Slope"=0.0}, {"X"=-1.1960255, "Y"=2.398121, "Slope"=0.0}, {"X"=-1.2145584, "Y"=2.405078, "Slope"=0.0}, {"X"=1.5076458, "Y"=1.9700412, "Slope"=0.0}, {"X"=1.78655, "Y"=1.4684, "Slope"=0.0}, {"X"=1.78655, "Y"=1.4684, "Slope"=0.0}, {"X"=1.8523945, "Y"=1.34997, "Slope"=0.0}, {"X"=1.8655576, "Y"=1.3262943, "Slope"=0.0}, {"X"=1.8931534, "Y"=1.2766625, "Slope"=0.0}, {"X"=1.8931534, "Y"=1.2766625, "Slope"=0.0}, {"X"=1.9770744, "Y"=1.1257194, "Slope"=0.0}, {"X"=1.9836459, "Y"=1.1138973, "Slope"=0.0}, {"X"=2.2579062, "Y"=0.62060535, "Slope"=0.0}, {"X"=2.3439512, "Y"=0.4658459, "Slope"=0.0}, {"X"=2.4375534, "Y"=0.29749277, "Slope"=0.0}, {"X"=2.4375534, "Y"=0.29749277, "Slope"=0.0}, {"X"=2.5186753, "Y"=0.151581, "Slope"=0.0}, {"X"=2.6968968, "Y"=-0.16897915, "Slope"=0.0}, {"X"=2.8735185, "Y"=-0.4866523, "Slope"=0.0}, {"X"=2.634508, "Y"=-0.056768816, "Slope"=0.0}, {"X"=2.8530045, "Y"=-0.44975382, "Slope"=0.0}, {"X"=1.1919955, "Y"=2.5377808, "Slope"=0.0}, {"X"=1.1919955, "Y"=2.5377808, "Slope"=0.0}, {"X"=1.5014237, "Y"=1.9812346, "Slope"=0.0}, {"X"=-1.4998013, "Y"=1.9812322, "Slope"=0.0}, {"X"=-1.5060034, "Y"=1.970079, "Slope"=0.0}, {"X"=-1.784904, "Y"=1.4684283, "Slope"=0.0}, {"X"=-1.857495, "Y"=1.3378601, "Slope"=0.0}, {"X"=-1.8507538, "Y"=1.3499885, "Slope"=0.0}, {"X"=-1.2245513, "Y"=2.476303, "Slope"=0.0}, {"X"=-1.0659869, "Y"=2.7614949, "Slope"=0.0}, {"X"=-1.7710594, "Y"=1.4933293, "Slope"=0.0}, {"X"=-1.8639268, "Y"=1.3262943, "Slope"=0.0}, {"X"=-1.8915226, "Y"=1.2766625, "Slope"=0.0}, {"X"=-1.9820136, "Y"=1.113902, "Slope"=0.0}, {"X"=-2.1730704, "Y"=0.7702549, "Slope"=0.0}, {"X"=-2.2562754, "Y"=0.62060535, "Slope"=0.0}, {"X"=-2.4359226, "Y"=0.29749277, "Slope"=0.0}, {"X"=-2.632877, "Y"=-0.056768816, "Slope"=0.0}, {"X"=-2.8513737, "Y"=-0.44975382, "Slope"=0.0}, {"X"=-2.3423204, "Y"=0.4658459, "Slope"=0.0}, {"X"=-2.5170445, "Y"=0.151581, "Slope"=0.0}, {"X"=-2.695266, "Y"=-0.16897915, "Slope"=0.0}, {"X"=-2.8718877, "Y"=-0.4866523, "Slope"=0.0}, {"X"=-1.9754436, "Y"=1.1257194, "Slope"=0.0}, {"X"=-6.1731024, "Y"=0.80225223, "Slope"=0.0}, {"X"=-6.4152503, "Y"=1.0218331, "Slope"=0.0}, {"X"=-6.608058, "Y"=1.2818588, "Slope"=0.0}, {"X"=-6.6882205, "Y"=1.5042956, "Slope"=0.0}, {"X"=-6.6324167, "Y"=1.8278004, "Slope"=0.0}, {"X"=-6.4458513, "Y"=2.1040184, "Slope"=0.0}, {"X"=-6.1973596, "Y"=2.3407633, "Slope"=0.0}, {"X"=-5.523589, "Y"=0.5446353, "Slope"=0.0}, {"X"=-5.79826, "Y"=2.4814765, "Slope"=0.0}, {"X"=-4.867923, "Y"=0.47854578, "Slope"=0.0}, {"X"=-5.3243194, "Y"=2.5744805, "Slope"=0.0}, {"X"=-3.50968, "Y"=1.0301466, "Slope"=0.0}, {"X"=-3.4327807, "Y"=1.2001191, "Slope"=0.0}, {"X"=-3.3941116, "Y"=1.382841, "Slope"=0.0}, {"X"=-3.4603047, "Y"=1.7814922, "Slope"=0.0}, {"X"=-4.809182, "Y"=0.48575115, "Slope"=0.0}, {"X"=-4.405914, "Y"=0.54676175, "Slope"=0.0}, {"X"=-4.595913, "Y"=2.5052567, "Slope"=0.0}, {"X"=-4.0831995, "Y"=0.6346704, "Slope"=0.0}, {"X"=-4.1484256, "Y"=2.3729658, "Slope"=0.0}, {"X"=-3.6613507, "Y"=0.885137, "Slope"=0.0}, {"X"=-3.85941, "Y"=0.7556109, "Slope"=0.0}, {"X"=-4.011697, "Y"=0.66795987, "Slope"=0.0}, {"X"=-6.1973596, "Y"=2.3407633, "Slope"=0.0}, {"X"=-5.79826, "Y"=2.4814765, "Slope"=0.0}, {"X"=-5.3243194, "Y"=2.5744805, "Slope"=0.0}, {"X"=-4.595913, "Y"=2.5052567, "Slope"=0.0}, {"X"=-6.4458513, "Y"=2.1040184, "Slope"=0.0}, {"X"=-3.5067923, "Y"=1.8703905, "Slope"=0.0}, {"X"=-3.5067923, "Y"=1.8703905, "Slope"=0.0}, {"X"=-6.6324167, "Y"=1.8278004, "Slope"=0.0}, {"X"=-3.4603047, "Y"=1.7814922, "Slope"=0.0}, {"X"=-6.6882205, "Y"=1.5042956, "Slope"=0.0}, {"X"=-3.3941116, "Y"=1.382841, "Slope"=0.0}, {"X"=-6.608058, "Y"=1.2818588, "Slope"=0.0}, {"X"=-3.4327807, "Y"=1.2001191, "Slope"=0.0}, {"X"=-6.4152503, "Y"=1.0218331, "Slope"=0.0}, {"X"=-3.50968, "Y"=1.0301466, "Slope"=0.0}, {"X"=-3.5353258, "Y"=0.9944994, "Slope"=0.0}, {"X"=-6.1731024, "Y"=0.80225223, "Slope"=0.0}, {"X"=-3.7040718, "Y"=0.85061496, "Slope"=0.0}, {"X"=-5.523589, "Y"=0.5446353, "Slope"=0.0}, {"X"=-4.405914, "Y"=0.54676175, "Slope"=0.0}, {"X"=-4.809182, "Y"=0.48575115, "Slope"=0.0}, {"X"=-4.1103888, "Y"=2.2329714, "Slope"=0.0}, {"X"=-4.869828, "Y"=2.4418511, "Slope"=0.0}, {"X"=-5.417605, "Y"=2.4471264, "Slope"=0.0}, {"X"=-5.843739, "Y"=2.3647609, "Slope"=0.0}, {"X"=-3.5717738, "Y"=1.6587385, "Slope"=0.0}, {"X"=-5.717605, "Y"=0.7264725, "Slope"=0.0}, {"X"=-6.403721, "Y"=1.1754698, "Slope"=0.0}, {"X"=-4.0733967, "Y"=2.213103, "Slope"=0.0}, {"X"=-4.0369825, "Y"=2.1945257, "Slope"=0.0}, {"X"=-3.8689134, "Y"=2.0467944, "Slope"=0.0}, {"X"=-3.8689134, "Y"=2.0467944, "Slope"=0.0}, {"X"=-3.695971, "Y"=1.8667909, "Slope"=0.0}, {"X"=-3.7373013, "Y"=1.9342899, "Slope"=0.0}, {"X"=-3.5643377, "Y"=1.6428626, "Slope"=0.0}, {"X"=-5.574709, "Y"=0.685647, "Slope"=0.0}, {"X"=-3.5498102, "Y"=1.3571969, "Slope"=0.0}, {"X"=-3.6723025, "Y"=1.0764607, "Slope"=0.0}, {"X"=-4.7639546, "Y"=0.60666454, "Slope"=0.0}, {"X"=-3.873783, "Y"=0.89096785, "Slope"=0.0}, {"X"=-4.470907, "Y"=0.6456365, "Slope"=0.0}, {"X"=-5.7393327, "Y"=2.4042227, "Slope"=0.0}, {"X"=-4.869828, "Y"=2.4418511, "Slope"=0.0}, {"X"=-5.417605, "Y"=2.4471264, "Slope"=0.0}, {"X"=-6.31894, "Y"=2.0987613, "Slope"=0.0}, {"X"=-6.31894, "Y"=2.0987613, "Slope"=0.0}, {"X"=-3.5643377, "Y"=1.6428626, "Slope"=0.0}, {"X"=-6.1827035, "Y"=0.97466177, "Slope"=0.0}, {"X"=-6.53032, "Y"=1.7503738, "Slope"=0.0}, {"X"=-6.3882627, "Y"=2.0303822, "Slope"=0.0}, {"X"=-3.5498102, "Y"=1.3571969, "Slope"=0.0}, {"X"=-6.5354886, "Y"=1.4654716, "Slope"=0.0}, {"X"=-6.53032, "Y"=1.7503738, "Slope"=0.0}, {"X"=-3.6723025, "Y"=1.0764607, "Slope"=0.0}, {"X"=-6.2342267, "Y"=1.0170529, "Slope"=0.0}, {"X"=-6.1827035, "Y"=0.97466177, "Slope"=0.0}, {"X"=-6.483632, "Y"=1.3510634, "Slope"=0.0}, {"X"=-3.717171, "Y"=1.0358701, "Slope"=0.0}, {"X"=-6.403721, "Y"=1.1754698, "Slope"=0.0}, {"X"=-6.3864765, "Y"=1.1548297, "Slope"=0.0}, {"X"=-6.0006623, "Y"=0.86890256, "Slope"=0.0}, {"X"=-5.574709, "Y"=0.685647, "Slope"=0.0}, {"X"=-4.470907, "Y"=0.6456365, "Slope"=0.0}, {"X"=-4.7639546, "Y"=0.60666454, "Slope"=0.0}, {"X"=-5.325075, "Y"=0.63066685, "Slope"=0.0}, {"X"=5.768352, "Y"=2.4869251, "Slope"=0.0}, {"X"=6.256812, "Y"=2.3057399, "Slope"=0.0}, {"X"=3.3904872, "Y"=1.4368991, "Slope"=0.0}, {"X"=6.115471, "Y"=0.7700497, "Slope"=0.0}, {"X"=4.9278536, "Y"=2.5646243, "Slope"=0.0}, {"X"=6.607655, "Y"=1.9358124, "Slope"=0.0}, {"X"=4.4356084, "Y"=2.454596, "Slope"=0.0}, {"X"=6.7040563, "Y"=1.5566156, "Slope"=0.0}, {"X"=4.024505, "Y"=2.3008115, "Slope"=0.0}, {"X"=6.6571274, "Y"=1.3635727, "Slope"=0.0}, {"X"=3.8814108, "Y"=2.2197797, "Slope"=0.0}, {"X"=6.5468025, "Y"=1.168247, "Slope"=0.0}, {"X"=3.4867268, "Y"=1.8398644, "Slope"=0.0}, {"X"=6.373358, "Y"=0.9706594, "Slope"=0.0}, {"X"=3.418811, "Y"=1.2466412, "Slope"=0.0}, {"X"=5.567228, "Y"=0.5589959, "Slope"=0.0}, {"X"=3.4960277, "Y"=1.0581442, "Slope"=0.0}, {"X"=3.6728444, "Y"=0.8732367, "Slope"=0.0}, {"X"=5.017665, "Y"=0.49480686, "Slope"=0.0}, {"X"=3.9657695, "Y"=0.6925165, "Slope"=0.0}, {"X"=4.5461817, "Y"=0.5221703, "Slope"=0.0}, {"X"=6.3164315, "Y"=0.9224521, "Slope"=0.0}, {"X"=3.474629, "Y"=1.8224995, "Slope"=0.0}, {"X"=3.4075844, "Y"=1.5070968, "Slope"=0.0}, {"X"=3.3904872, "Y"=1.4368991, "Slope"=0.0}, {"X"=5.517816, "Y"=0.5428311, "Slope"=0.0}, {"X"=4.866611, "Y"=0.4799412, "Slope"=0.0}, {"X"=5.567228, "Y"=0.5589959, "Slope"=0.0}, {"X"=4.210116, "Y"=0.57917607, "Slope"=0.0}, {"X"=6.115471, "Y"=0.7700497, "Slope"=0.0}, {"X"=6.1346426, "Y"=0.7791764, "Slope"=0.0}, {"X"=3.9657695, "Y"=0.6925165, "Slope"=0.0}, {"X"=6.373358, "Y"=0.9706594, "Slope"=0.0}, {"X"=3.543388, "Y"=0.9885701, "Slope"=0.0}, {"X"=6.5468025, "Y"=1.168247, "Slope"=0.0}, {"X"=3.4960277, "Y"=1.0581442, "Slope"=0.0}, {"X"=6.6571274, "Y"=1.3635727, "Slope"=0.0}, {"X"=3.418811, "Y"=1.2466412, "Slope"=0.0}, {"X"=6.7040563, "Y"=1.5566156, "Slope"=0.0}, {"X"=6.607655, "Y"=1.9358124, "Slope"=0.0}, {"X"=3.514335, "Y"=1.8804414, "Slope"=0.0}, {"X"=6.111094, "Y"=2.3925397, "Slope"=0.0}, {"X"=5.4517217, "Y"=2.575982, "Slope"=0.0}, {"X"=4.7988167, "Y"=2.5636787, "Slope"=0.0}, {"X"=4.1516795, "Y"=2.3743773, "Slope"=0.0}, {"X"=3.8814108, "Y"=2.2197797, "Slope"=0.0}, {"X"=3.9731412, "Y"=0.83052903, "Slope"=0.0}, {"X"=3.795828, "Y"=0.9617485, "Slope"=0.0}, {"X"=3.6591375, "Y"=1.1025287, "Slope"=0.0}, {"X"=3.5967474, "Y"=1.7109286, "Slope"=0.0}, {"X"=4.601434, "Y"=2.407352, "Slope"=0.0}, {"X"=4.247952, "Y"=0.71311134, "Slope"=0.0}, {"X"=4.5937724, "Y"=0.6193031, "Slope"=0.0}, {"X"=6.360058, "Y"=2.0599158, "Slope"=0.0}, {"X"=6.473898, "Y"=1.8649976, "Slope"=0.0}, {"X"=6.534187, "Y"=1.6240577, "Slope"=0.0}, {"X"=6.438916, "Y"=1.2494335, "Slope"=0.0}, {"X"=6.352519, "Y"=1.1123196, "Slope"=0.0}, {"X"=6.1843343, "Y"=0.97466177, "Slope"=0.0}, {"X"=5.7946186, "Y"=0.74757576, "Slope"=0.0}, {"X"=5.7946186, "Y"=0.74757576, "Slope"=0.0}, {"X"=6.473898, "Y"=1.8649976, "Slope"=0.0}, {"X"=4.8706145, "Y"=2.4416611, "Slope"=0.0}, {"X"=5.4187417, "Y"=2.447126, "Slope"=0.0}, {"X"=5.100068, "Y"=0.6077611, "Slope"=0.0}, {"X"=5.2293944, "Y"=0.60893834, "Slope"=0.0}, {"X"=5.5763397, "Y"=0.685647, "Slope"=0.0}, {"X"=4.5937724, "Y"=0.6193031, "Slope"=0.0}, {"X"=4.247952, "Y"=0.71311134, "Slope"=0.0}, {"X"=4.084907, "Y"=0.7651222, "Slope"=0.0}, {"X"=3.5614526, "Y"=1.3278108, "Slope"=0.0}, {"X"=3.5644014, "Y"=1.6208274, "Slope"=0.0}, {"X"=3.8754106, "Y"=0.89096767, "Slope"=0.0}, {"X"=6.5370927, "Y"=1.4654024, "Slope"=0.0}, {"X"=3.5614526, "Y"=1.3278108, "Slope"=0.0}, {"X"=3.6739268, "Y"=1.0764607, "Slope"=0.0}, {"X"=3.5514364, "Y"=1.3571784, "Slope"=0.0}, {"X"=6.534187, "Y"=1.6240577, "Slope"=0.0}, {"X"=3.5967474, "Y"=1.7109286, "Slope"=0.0}, {"X"=6.138734, "Y"=2.2173433, "Slope"=0.0}, {"X"=5.845225, "Y"=2.3647902, "Slope"=0.0}, {"X"=4.0386133, "Y"=2.1945257, "Slope"=0.0}, {"X"=4.0386133, "Y"=2.1945257, "Slope"=0.0}, {"X"=6.360058, "Y"=2.0599158, "Slope"=0.0}, {"X"=6.320571, "Y"=2.0987613, "Slope"=0.0}, {"X"=4.8706145, "Y"=2.4416611, "Slope"=0.0}, {"X"=5.4187417, "Y"=2.447126, "Slope"=0.0}, {"X"=6.0050135, "Y"=2.3015885, "Slope"=0.0}]}, "VertexArray"=w10) -> (→"Poly2D":T1)
